vi "CRYStimulus Editor.vi"() -> ()   [LabVIEW 2013]
uses:
  <vilib>/Utility/miscctls.llb/LVBoundsTypeDef.ctl
  Typedef Control/CRYStimulus Cluster.ctl
  Typedef Control/CRYHardware Channel Info.ctl
  Control/CRYStimulusGraphWave.ctl
  CRYProject/CRYProject Editor Global.vi
  SubVI/CRYStimulus Global.vi
  CRYMainGlobal.vi
  CRYWindow/SubVI/CRYMain Sub Window Global.vi
  Program/CRYRef nums global.vi
  CRYStepSetup/CRYStepSetup Global.vi
  CRYSound.dll
panel:
  in  "OkCancelClicked":bool caption="Apply"
  out "Stimulus Bk":T1={"StimulusType"="", "UseMLValArray"=[], "ML_axisArray"=[], "MLValLevelNameArray"=[], "Level(U)Array"=[1.0, 0.0, 0.0, 0.0, 0.0, 0.0, 0.26], "Start(Stop)FreqArray"=[20000.0, 20.0], "Start(Stop)AmpArray"=[0.5, 1.0], "StepResolutionArray"=[], "Unit_Array"=[], "DegValArray"=[], "DegUnitArray"=[], "Steps1"=19, "Cycle/step1(#)"=20, "Time/step1(s)"=0.01, "Transition1"=0.0, "SweepRate2"=1.0, "Freq3(Hz)"=0.0, "Steps3(#)"=19.0, "Cycles3(#)"=12, "StepSize3"=0.0, "wave time"="", "RMS_Value4"=0.0, "Peak_Value4"=0.0, "WavePath4"="", "RMS_unit4"="", "Peak_unit4"="", "wave Info"="", "dc_ctrl5_1"=0, "dc_ctrl5_2"=0, "dc_polar5"=0, "Max.Current"=0, "Steps5(#)"=19, "Time/Step5"=0.05, "Level5"=0.0, "StepsSize5Val"=0.0, "StepSize5Unit"="", "SweepType"=0, "Fixed/Ratio6"=0, "Transition6"=0.0, "Steps6(#)"=19.0, "Cycle/Steps6(#)"=12, "Time/Steps6(s)"=0.0, "Freq6(Hz)"=0.0, "Difference6(Hz)"=0.0, "Ratio6"="", "NoiseType7"=0, "Duration7(s)"=1.0, "MinFreq7(Hz)"=20000.0, "MaxFreq7(Hz)"=20.0, "MinFreq8(Hz)"=20000.0, "MaxFreq8(Hz)"=20.0, "FreqRounding8"=FALSE, "Duration8(s)"=1.0, "Tones8"=0.0, "RoundingVal8"=0.0, "ApplyEQ"=FALSE, "Duration(s)"=0.0, "CustomStimulusName "="", "Flatten Element Array"=[], "sine waves"=[], "Channel Out"=0, "RatioVal6"=0.0, "TabCtrl6"=enum."Master Tone", "Signal Type Name"="", "Help"="", "Channel Sel"=19, "V on DUT"=FALSE, "Output Imp"=6300.0, "Nominal Imp"=100.0} {"Nominal Imp" format="%.2p"; "Output Imp" format="%.2p"; "sine waves"."cycles" format="%.2f"; "sine waves"."ampl" format="%.2f"; "sine waves"."freq" format="%.2f"}
  in  "UpdateTemp":bool caption="Update"
  in  "CurLibChange":bool caption="Add Lib"
  in  "Buffer Index":u32
  in  "Device Name":string
  in  "Asio Limit":u32=16
  in  "Asio Inited":bool caption="Update"
  in  "Audio Driver":u16=16
  in  "Add Lib":bool
  in  "AddStep":bool
  out "Sens Value":dbl
  in  "Help Change":string
  out "EndFlag":bool
  out "Stimulus Play Wave":sgl[](array[numeric])
  out "Is Change?":bool
  in  "Curve Change":enum16{"Curves", "Values", "Results", "WFM"}[](array[ring])
  in  "Channel Out":u32=16
  out "Proper VI No":i32
  out "Signal Type Name":string
  in  "Is First":bool
  in  "Is SubPan?":bool
  out "O_channel Info Out":T2[](array[typedef]) {"Coupling" items=["Default"=-1, "RSE"=10083, "NRSE"=10078, "Differential"=10106, "Pseudodifferential"=12529]; "term config" items=["Default"=-1, "RSE"=10083, "NRSE"=10078, "Differential"=10106, "Pseudodifferential"=12529]; "Anti-aliasing Factor (%fs)" format="%.2f"}
  in  "Vp Out":dbl=2.6 min=0.1 step=0.01 format="%.2f"
  in  "Fs":u32=44100
  in  "BitDepth":u32=16
  in  "Output Device":i16
  in  "ntaskID":u32
  out "Stimulus Wave":sgl[](array[numeric])
  in  "Flatten Element Array":string[](array[string])
  in  "Load Test":bool
  out "Stimulus":T1={"StimulusType"="", "UseMLValArray"=[], "ML_axisArray"=[], "MLValLevelNameArray"=[], "Level(U)Array"=[1.0, 0.0, 0.0, 0.0, 0.0, 0.0, 0.26], "Start(Stop)FreqArray"=[20000.0, 20.0], "Start(Stop)AmpArray"=[0.5, 1.0], "StepResolutionArray"=[], "Unit_Array"=[], "DegValArray"=[], "DegUnitArray"=[], "Steps1"=19, "Cycle/step1(#)"=20, "Time/step1(s)"=0.01, "Transition1"=0.0, "SweepRate2"=1.0, "Freq3(Hz)"=0.0, "Steps3(#)"=19.0, "Cycles3(#)"=12, "StepSize3"=0.0, "wave time"="", "RMS_Value4"=0.0, "Peak_Value4"=0.0, "WavePath4"="", "RMS_unit4"="", "Peak_unit4"="", "wave Info"="", "dc_ctrl5_1"=0, "dc_ctrl5_2"=0, "dc_polar5"=0, "Max.Current"=0, "Steps5(#)"=19, "Time/Step5"=0.05, "Level5"=0.0, "StepsSize5Val"=0.0, "StepSize5Unit"="", "SweepType"=0, "Fixed/Ratio6"=0, "Transition6"=0.0, "Steps6(#)"=19.0, "Cycle/Steps6(#)"=12, "Time/Steps6(s)"=0.0, "Freq6(Hz)"=0.0, "Difference6(Hz)"=0.0, "Ratio6"="", "NoiseType7"=0, "Duration7(s)"=1.0, "MinFreq7(Hz)"=20000.0, "MaxFreq7(Hz)"=20.0, "MinFreq8(Hz)"=20000.0, "MaxFreq8(Hz)"=20.0, "FreqRounding8"=FALSE, "Duration8(s)"=1.0, "Tones8"=0.0, "RoundingVal8"=0.0, "ApplyEQ"=FALSE, "Duration(s)"=0.0, "CustomStimulusName "="", "Flatten Element Array"=[], "sine waves"=[], "Channel Out"=0, "RatioVal6"=0.0, "TabCtrl6"=enum."Master Tone", "Signal Type Name"="", "Help"="", "Channel Sel"=19, "V on DUT"=FALSE, "Output Imp"=6300.0, "Nominal Imp"=100.0} {"Nominal Imp" format="%.2p"; "Output Imp" format="%.2p"; "sine waves"."cycles" format="%.2f"; "sine waves"."ampl" format="%.2f"; "sine waves"."freq" format="%.2f"}
  in  "All Parameter Change":bool
  out "VIMiniumBound":T3
  in  "Channel":i32
  in  "Calibration setup In":string
  in  "Hardware setup In":string
  out "Flatten Stimulus Out":string
  in  "reference out":refnum<vi>
  in  "stop":bool
  in  "Board Tab":enum32{"Page 1"}(tab) caption="Control Tab"
  in  "Progress":string
  in  "Apply EQ":bool caption="使用均衡器"
  in  "Custom Stimulus Name":string caption="自定义激励名称"
  out "Duration(s)":dbl caption="持续时间(s)" format="%#_6p"
  in  "Update":bool
  in  "Play":bool
  in  "Output Channel":bool
  in  "ViewTable":bool
  in  "Table Tab":enum32{"Setting", "Help"}(tab)
  in  "Move Down":bool
  in  "Move Up":bool
  in  "Remove":bool
  in  "Insert":bool
  in  "Edit":bool
  in  "Multicolumn Listbox":i32(listbox)
  in  "Help":string
  in  "delta_str":string
  in  "delta_X":dbl format="%#.3p"
  in  "delta_Y":dbl
  in  "View Edit":bool
  out "Wave graph":T4
  in  "Buf Amount":u32=16
  out "Stim max value":sgl
  in  "Revert":bool caption="Apply"
  in  "Load...":bool caption="Apply"
  in  "Save As...":bool caption="Apply"
  in  "OK":bool caption="Apply"
  in  "Cancel":bool caption="Apply"
  # "(1,2,3,4,6_1,6_2,7,8)"
  # "(1,2,3,4,6_1,6_2,7,8)"
  # "(1,2,3,4,6_1,6_2,7,8)"
  # "(1,2,4,6_1,6_2,7,8)"
  # "(1,2,6)"
  # "(3,5)"
  # "(1,6,8)"
  # "(1,2,4,6_1,6_2,7,8)"
  # "(1,2,3,4,6_1,6_2,7,8)"
  # "(1,2,3,4,6_1,6_2,7,8)"
  # "(1,2,3,4,6_1,6_2,7,8)"
  # "(1,2,3,4,6_1,6_2,7,8)"
  # "(1,2,3,4,6_1,6_2,7,8)"
  # "(1,2,4,6_1,6_2,7,8)"
  # "(1,2,6)"
  # "(3,5)"
  # "(1,6,8)"
  # "(1,2,4,6_1,6_2,7,8)"
  # "(1,2,3,4,6_1,6_2,7,8)"
  # "(1,2,3,4,6_1,6_2,7,8)"
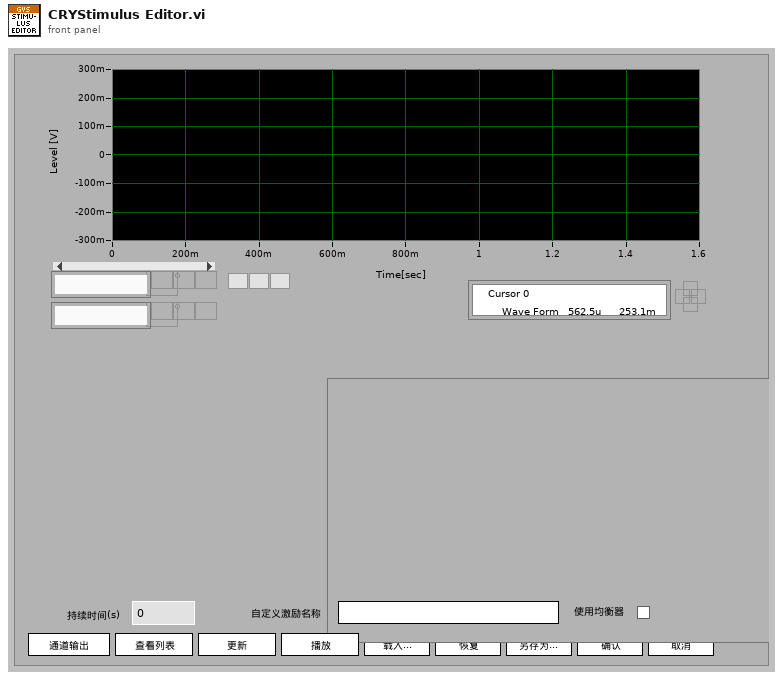
[diagram p1: front panel]
types:
  T1 = typedef "CRYStimulus Cluster.ctl" = cluster{"StimulusType":string, "UseMLValArray":u16[], "ML_axisArray":u16[], "MLValLevelNameArray":string[], "Level(U)Array":dbl[], "Start(Stop)FreqArray":dbl[], "Start(Stop)AmpArray":dbl[], "StepResolutionArray":u16[], "Unit_Array":u16[], "DegValArray":dbl[], "DegUnitArray":string[], "Steps1":i32, "Cycle/step1(#)":u32, "Time/step1(s)":dbl, "Transition1":dbl, "SweepRate2":dbl, "Freq3(Hz)":dbl, "Steps3(#)":dbl, "Cycles3(#)":u32, "StepSize3":dbl, "wave time":string, "RMS_Value4":dbl, "Peak_Value4":dbl, "WavePath4":string, "RMS_unit4":string, "Peak_unit4":string, "wave Info":string, "dc_ctrl5_1":u16, "dc_ctrl5_2":u16, "dc_polar5":u16, "Max.Current":u16, "Steps5(#)":u32, "Time/Step5":dbl, "Level5":dbl, "StepsSize5Val":dbl, "StepSize5Unit":string, "SweepType":u16, "Fixed/Ratio6":u16, "Transition6":dbl, "Steps6(#)":dbl, "Cycle/Steps6(#)":u32, "Time/Steps6(s)":dbl, "Freq6(Hz)":dbl, "Difference6(Hz)":dbl, "Ratio6":string, "NoiseType7":u16, "Duration7(s)":dbl, "MinFreq7(Hz)":dbl, "MaxFreq7(Hz)":dbl, "MinFreq8(Hz)":dbl, "MaxFreq8(Hz)":dbl, "FreqRounding8":bool, "Duration8(s)":dbl, "Tones8":dbl, "RoundingVal8":dbl, "ApplyEQ":bool, "Duration(s)":dbl, "CustomStimulusName ":string, "Flatten Element Array":string[], "sine waves":cluster{"freq":dbl, "ampl":dbl, "cycles":dbl}[], "Channel Out":i32, "RatioVal6":dbl, "TabCtrl6":enum32{"Master Tone", "Slave Tone"}, "Signal Type Name":string, "Help":string, "Channel Sel":u16, "V on DUT":bool, "Output Imp":dbl, "Nominal Imp":dbl}
  T2 = typedef "CRYHardware Channel Info.ctl" = cluster{"ID":i32, "Name":string, "Digital":bool, "Input":bool, "Device Name":string, "Hardware Ch ID":u8, "Vmax (V)":dbl, "Latency (samples)":dbl, "Sampling Rate (Hz)":u32, "Bit Depth":u32, "Anti-aliasing Factor (%fs)":sgl, "DAQmx Channel":tag, "term config":i32, "Coupling":i32, "IEPE en":bool, "ASIOChannel Name":string, "Audio Driver":u16, "ASIOChannel Index":u8}
  T3 = typedef "LVBoundsTypeDef.ctl" = cluster{"Width":u32, "Height":u32}
  T4 = typedef "CRYStimulusGraphWave.ctl" = waveform(dbl)
  T5 = cluster{"halt now":bool, "exit":bool, "dll done":bool, "Hardware":i32, "start":bool}
  T6 = typedef "CRYHardware.ctl" = cluster{"Name":string, "Analog I/O":u16, "Digital I/O":u16, "Channels":u8, "Dig Dev ID":u8, "N ports":u8, "Interface":u32, "Dig I/O Ports":cluster{"port #":i16, "width":i16, "direction":i32}[], "Interf settings":cluster{"Type":u16, "COM Port":u8, "Baud rate":u32, "Data bits":u32, "Parity":u16, "Stop bits":u16, "Flow control":u16, "Dev ID IEEE":u8}[], "N interfs":i32, "udev SNs":i16[], "udev enable":bool, "Channel Array":T2[], "Cal sequence":string, "SelectedIn":u16, "SelectedOut":u16, "SelectedTab":u16, "State":bool, "Help":string, "Advanced":bool, "In Audio Driver":u16, "Out Audio Driver":u16}
  T7 = typedef "CRYCalibration All Cluster.ctl" = cluster{"Calibration 2D":T8[], "Help":string, "Tab Value":i32, "Input Signal Type":string, "Output Signal Type":string}
  T8 = typedef "CRYCalibration 2DCluster.ctl" = cluster{"Calibration":T9, "Corr Curve":T10, "EQ Curve":T10, "Sens Curve":T10}
  T9 = typedef "CRYCalibration Cluster.ctl" = cluster{"Calibration Step Name":string, "Device":string, "Correction Curve Name":string, "Equalization Curve Name":string, "Sensitivity Curve Name":string, "Corr Folder and File":string, "EQ Folder and File":string, "Sens Folder and File":string, "Corr Step size":u16, "EQ Step size":u16, "Input":bool, "Last Cal Date (sec)":timestamp, "Cha Name":string, "Corr Curve Found":bool, "EQ Curve Found":bool, "Sens Curve Found":bool, "Signal Type":string, "Calibrated Device":string, "Hz":u32}
  T10 = typedef "CRYData Cluster.ctl" = cluster{"Name":string, "Curve":cluster{"x":dbl, "y":dbl, "z":dbl}[], "X data":u16, "Y data":u16, "Z data":u16, "X axis":u16, "Y axis":u16, "Z axis":u16, "X unit":string, "Y unit":string, "Z unit":string, "X dB ref":dbl, "Y dB ref":dbl, "Z dB ref":dbl, "single val":bool, "protected":bool, "display X":bool, "display Y":bool, "display Z":bool, "Test Info":string, "Step No.":i32, "Plot Settings":cluster{"Color":u32, "Interpolation":u8, "Point Style":u8, "Line Style":u8, "Point Color":u32, "Line Width":u8, "Bar Plot Style":u8, "Fill To":i16}, "AutoProtect":bool}
  T11 = typedef "CRYStep.ctl" = cluster{"No.VI":i32, "Category":string, "StepName":string, "Seq setup flattened":string, "Comment":string, "Steps config.":bool[], "Jump config":i32[], "Start":dbl, "Increment":dbl, "Name":string, "Unit":string, "Y data":u16, "Y prefix":string, "Y dB ref":dbl, "Y unit":string, "Repeat State Array":cluster{"Start":dbl, "Increment":dbl, "Count":i32, "Num":i32}[]}
  T12 = enum8{"Enabled", "Disabled", "Disabled and Grayed Out"}
  T13 = enum32{"Invalid", "Default", "Floating", "Floating/Auto-Hide", "Modal"}
  T14 = enum16{"OK", "Yes", "YesNo", "YesNoCancel", "ReplaceAppend"}
  T15 = typedef "CRYWaveform Cluster.ctl" = cluster{"Waveform":cluster{"X0":dbl, "dX":dbl, "Y":sgl[]}, "X data":u16, "Y data":u16, "Y axis":u16, "X unit":string, "Y unit":string, "Y dB ref":dbl, "display Y":bool, "display X":bool, "Overload?":bool, "Test Info":string, "Step No.":i32, "Name":string, "protected":bool, "Sqc history":string[], "Signal Channel ID":i32, "Plot Settings":cluster{"Color":u32, "Interpolation":u8, "Point Style":u8, "Line Style":u8, "Point Color":u32, "Line Width":u8, "Bar Plot Style":u8, "Fill To":i16}, "AutoProtect":bool}
  T16 = cluster{"Load Test":bool, "Output Channel":bool, "Edit":bool, "Insert":bool, "Remove":bool, "Move Up":bool, "Move Down":bool, "ViewTable":bool, "View Edit":bool, "Add Lib":bool, "OK":bool, "Cancel":bool}
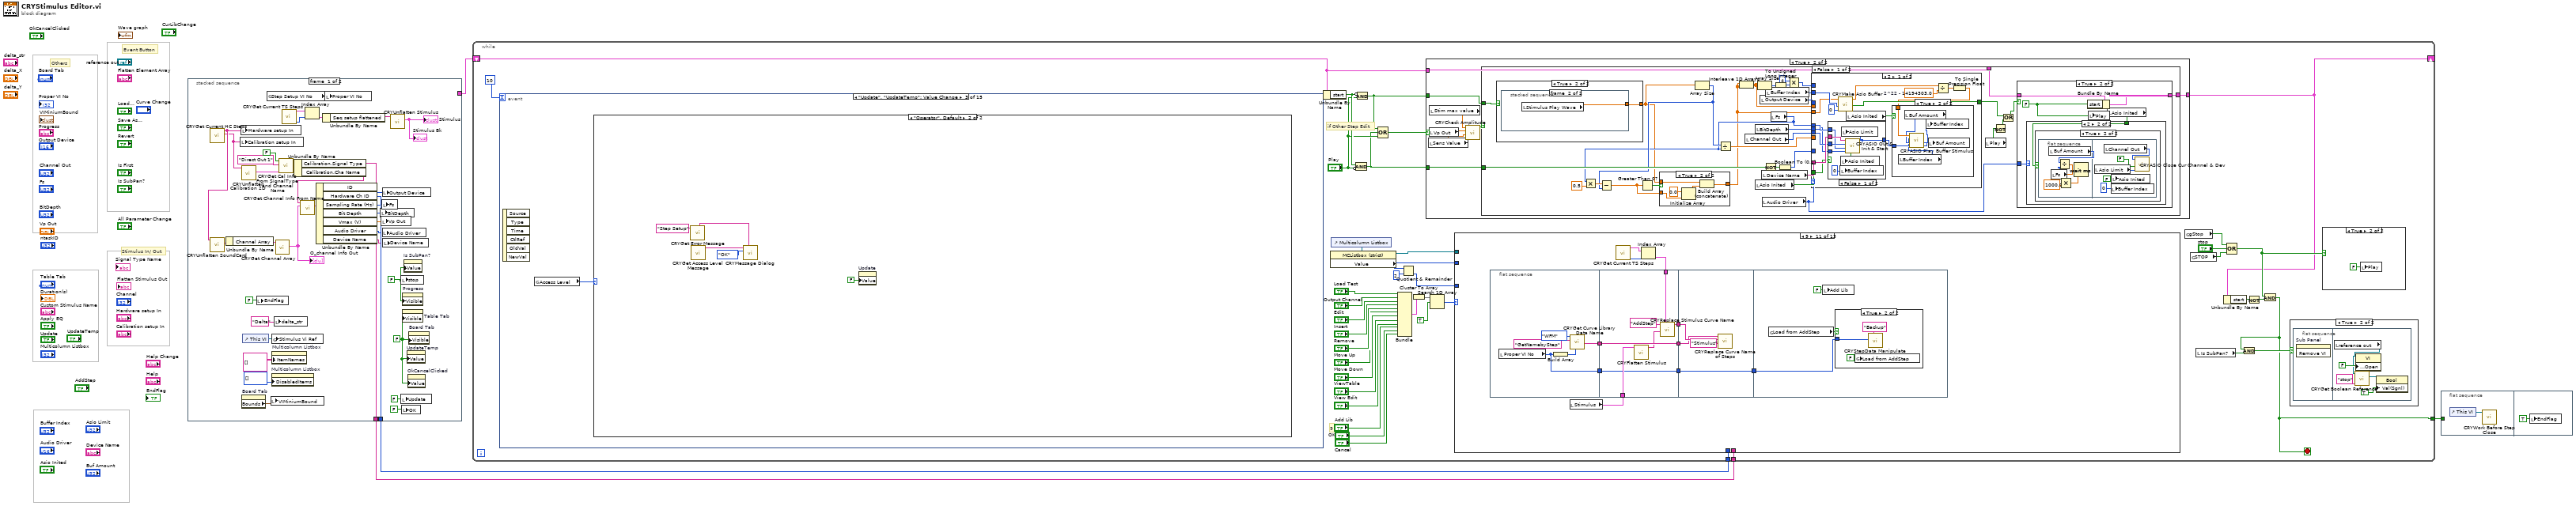
[diagram p0: block diagram]
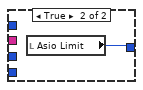
[diagram p6: hidden frame]
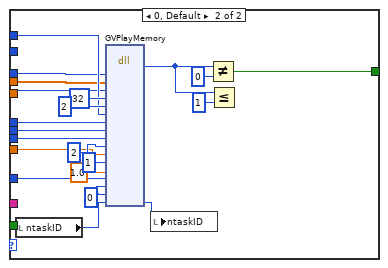
[diagram p7: hidden frame]
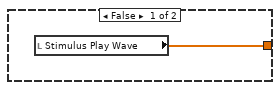
[diagram p9: hidden frame]
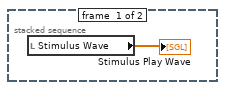
[diagram p10: hidden frame]
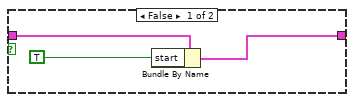
[diagram p11: hidden frame]
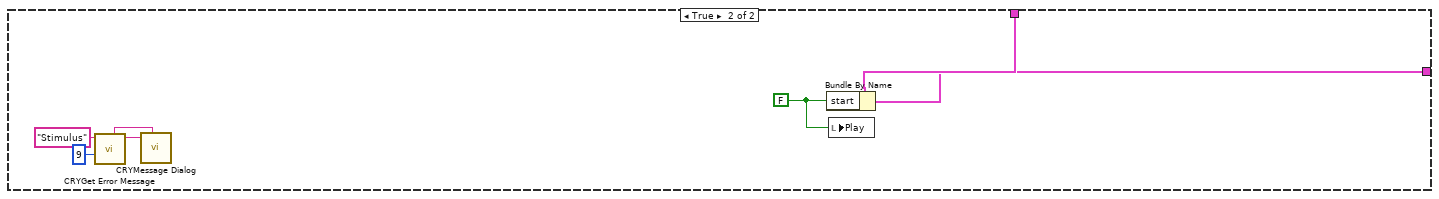
[diagram p14: hidden frame]
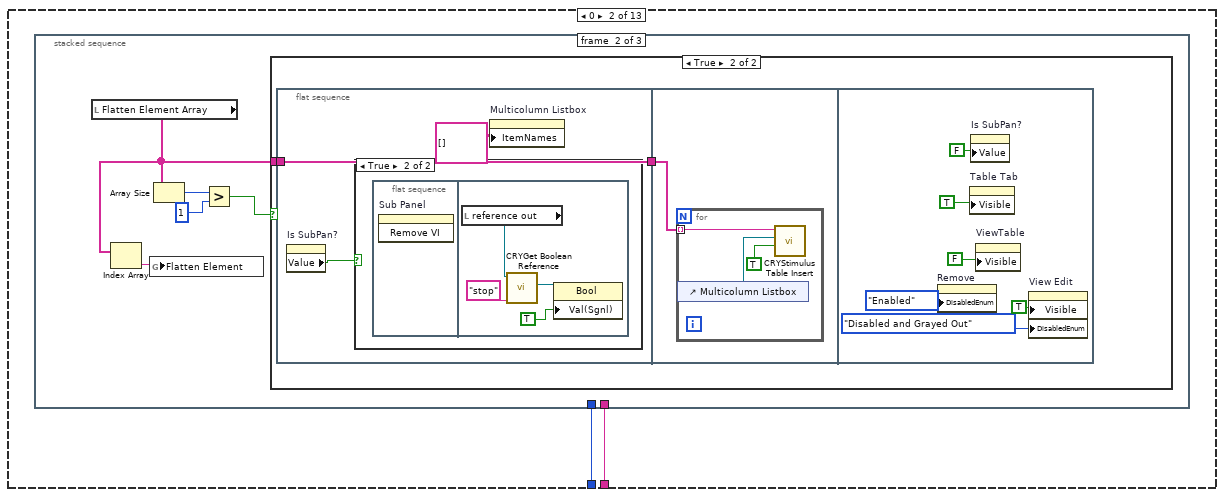
[diagram p16: hidden frame]
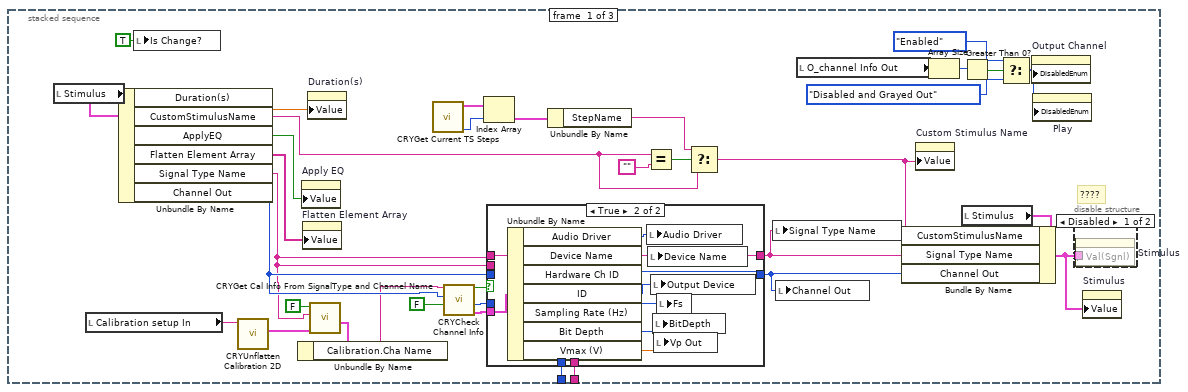
[diagram p17: hidden frame]
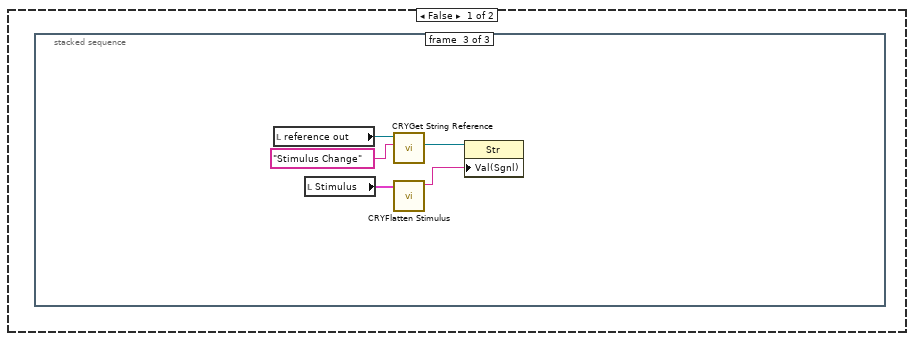
[diagram p20: hidden frame]
diagram:
  # "Others"
  # "Event Button"
  # "Stimulus In/ Out"
  n1 = stacked-sequence {
    tunnel: [_ T5 {"halt now"=FALSE, "exit"=FALSE, "dll done"=FALSE, "Hardware"=-1, "start"=FALSE}] -> w4
    tunnel: [w14 _] -> w2
    tunnel: [w23 _] -> w3
    frame #0 {
      w7 = FALSE ("Visible")
      w27 = FALSE ("Visible")
      n2 = call "CRYGet Current HC Steps.vi"() -> ("Calibration setup flattened Out"=w19:string, "Hardware setup flattened Out"=w20:string)  [unwired: 10 in]
      n3 = call "CRYUnflatten SoundCard.vi"("Flatten SoundCard"=w20) -> ("SoundCard"=w33:T6)  [unwired: 10 out]
      n4 = Unbundle By Name(w33) -> ("Channel Array"=w34:T2[])
      n5 = local write "Calibration setup In"(w19) -> ()
      n6 = local write "Hardware setup In"(w20) -> ()
      n7 = call "CRYUnflatten Calibration 2D.vi"("Flattened Calibration"=w19) -> ("Calibration Step Out"=w18:T7)  [unwired: 8 in, 2 out]
      n8 = property on="Board Tab" class="TabCtl (strict)"() -> ("Bounds"=w38:T3)  [unwired: 2 in, 2 out]
      n9 = control-ref of="This VI"() -> (w28:refnum<vi>)
      n10 = local write "EndFlag"(FALSE ("endflag")) -> ()
      n11 = global read "CRYProject Editor Global.vi" "Step Setup VI No"() -> (w39:i32)
      n12 = local write "VIMiniumBound"(w38) -> ()
      n13 = global write "CRYStimulus Global.vi" "Stimulus Vi Ref"(w28) -> ()
      n14 = property on="Multicolumn Listbox" class="MCListbox (strict)"("DisabledItems"=i32[] [] ("Disabled Items")) -> ()  [unwired: 2 in, 2 out]
      n15 = property on="Multicolumn Listbox" class="MCListbox (strict)"("ItemNames"=string[][] [] ("Item Names")) -> ()  [unwired: 2 in, 2 out]
      n16 = local write "delta_str"("Delta" ("delta_str")) -> ()
      n17 = call "CRYGet Channel Array.vi"("Channel Array"=w34) -> ("O Channel Info Out"=w13:T2[])  [unwired: 10 out]
      "O_channel Info Out" <- w13
      n18 = call "CRYGet Cal Info From SignalType and Channel Name.vi"("Calibration"=w18, "Signal Type"="Direct Out 1" ("Calibration.Signal Type"), "In/Out?"=FALSE) -> ("Calibration 2D Cluster"=w15:T8)  [unwired: 6 in, 2 out]
      n19 = call "CRYGet Current TS Steps.vi"() -> ("SelectStepNumber in Tree"=w25:i32, "Steps"=w26:T11[])  [unwired: 1 in, 9 out]
      n20 = Unbundle By Name(w15) -> ("Calibration.Signal Type"=w14:string, "Calibration.Cha Name"=w12:string)
      n21 = call "CRYGet Channel Info From Name.vi"("Channel Info Array In"=w13, "Channel Name"=w12) -> ("ChannelInfo"=w11:T2)  [unwired: 8 in, 1 out]
      n22 = Index Array(array=w26, index=w25) -> (element=w35:T11)
      n23 = Unbundle By Name(w11) -> ("ID"=w29:i32, "Hardware Ch ID"=w23:u8, "Sampling Rate (Hz)"=w30:u32, "Bit Depth"=w32:u32, "Vmax (V)"=w31:dbl, "Audio Driver"=w10:u16, "Device Name"=w9:string)
      n24 = Unbundle By Name(w35) -> ("Seq setup flattened"=w36:string)
      n25 = local write "Proper VI No"(w39) -> ()
      n26 = local write "BitDepth"(w32) -> ()
      n27 = local write "Vp Out"(w31) -> ()
      n28 = local write "Fs"(w30) -> ()
      n29 = local write "Output Device"(w29) -> ()
      n30 = local write "Audio Driver"(w10) -> ()
      n31 = local write "Device Name"(w9) -> ()
      n32 = call "CRYUnflatten Stimulus.vi"("Flatten Stimulus"=w36) -> ("Stimulus"=→"Stimulus" →"Stimulus Bk":T1)  [unwired: 10 out]
      n33 = local write "stop"(w27) -> ()
      n34 = local write "Update"(FALSE ("Update")) -> ()
      n35 = local write "OK"(FALSE ("OK")) -> ()
      n36 = property on="Table Tab" class="TabCtl (strict)"("Visible"=w7) -> ()  [unwired: 2 in, 2 out]
      n37 = property on="Progress" class="Str"("Visible"=w27) -> ()  [unwired: 2 in, 2 out]
      n38 = property on="Is SubPan?" class="Bool (strict)"("Value"=w27) -> ()  [unwired: 2 in, 2 out]
      n39 = property on="UpdateTemp" class="Bool (strict)"("Value"=w7) -> ()  [unwired: 2 in, 2 out]
      n40 = property on="OkCancelClicked" class="Bool (strict)"("Value"=w7) -> ()  [unwired: 2 in, 2 out]
      n41 = property on="Board Tab" class="TabCtl (strict)"("Visible"=w7) -> ()  [unwired: 2 in, 2 out]
    }
    frame #1 {
      w41 = TRUE ("Load Test")
      n42 = local write "Stimulus Play Wave"(sgl[] [] ("Stimulus Play Wave")) -> ()
      n43 = local write "Is Change?"(w41) -> ()
      n44 = local write "Load Test"(w41) -> ()
      n45 = property on="Is First" class="Bool (strict)"("Value"=w41) -> ()  [unwired: 2 in, 2 out]
    }
  }
  n46 = while {
    shift-right: [w45] -> _
    shift-left: w4 -> [w75]
    tunnel: w3 -> [w52]
    tunnel: w2 -> [w53]
    tunnel: [w48] -> w1
    stop <- w48 stop-if-true
    # "9"
    # "if Other Step Edit"
    n47 = event shown="[2] \"Update\", \"UpdateTemp\": Value Change" {
      selector: _ -> [_ _ _ _ _ _ _ _ _ _ _ _ _ _ _]
      dyn-events: _ -> [_ _ _ _ _ _ _ _ _ _ _ _ _ _ _]
      timeout: 10 -> [_ _ _ _ _ _ _ _ _ _ _ _ _ _ _]
      event Timeout {
        n48 = event-data() -> ()  [unwired: 3 out]
      }
      event Pane Size {
        n49 = event-data() -> ()  [unwired: 7 out]
        n50 = control-ref of="Board Tab"() -> (w673:refnum<vi>)
        n51 = control-ref of="This VI"() -> (w674:refnum<vi>)
        n52 = call "CRYAlign Steps VI Center.vi"("Tab2"=w673, "Input/Output"=TRUE, "VIRef"=w674) -> ()  [unwired: 1 in, 8 out]
      }
      event "Update", "UpdateTemp": Value Change {
        n53 = event-data() -> ()  [unwired: 7 out]
        n54 = global read "CRYMainGlobal.vi" "Access Level"() -> (w676:enum16{"Engineer", "Technician", "Operator"})
        n55 = case shown="\"Operator\", Default" w676 {
          frame "Engineer" {
            n56 = property on="Table Tab" class="TabCtl (strict)"() -> ("Visible"=w678:bool)  [unwired: 2 in, 2 out]
            n57 = property on="Is First" class="Bool (strict)"() -> ("Value"=w679:bool)  [unwired: 2 in, 2 out]
            n58 = case shown="False" w678 {
              tunnel: w679 -> [w681 _]
              tunnel: [w680 w705] -> w677
              frame False {
                n59 = case shown="False" w681 {
                  tunnel: [w685 TRUE ("Error")] -> w680
                  frame False {
                    w690 = TRUE ("Is SubPan?")
                    n60 = local read "Flatten Element Array"() -> (w688:string[])
                    n61 = global read "CRYStimulus Global.vi" "Flatten Element"() -> (w689:string)
                    n62 = local read "Is Change?"() -> (w683:bool)
                    n63 = Index Array(array=w688) -> (element=w687:string)  [unwired: 1 in]
                    n64 = call "CRYCheck Change Before Update.vi"("New Flatten Stimulus Element"=w689, "Old Flatten Stimulus Element"=w687) -> ("Is Change?"=w684:bool)  [unwired: 9 out]
                    n65 = call "CRYCheck EditVal.vi"("Is SubPan?"=w690, "display message?"=w690, "Flatten Element"=w689) -> ("Error"=w686:bool)  [unwired: 1 in, 7 out]
                    n66 = Or(x=w684, y=w683) -> (x .or. y?=w682:bool)
                    n67 = Compound Arithmetic op=AND(invert w686, w682) -> (w685:bool)
                    n68 = case shown="True" w685 {
                      tunnel: w689 -> [_ w692]
                      tunnel: w688 -> [_ w691]
                      frame False {
                      }
                      frame True {
                        n69 = Array Size(array=w691) -> (size(s)=w695:i32)
                        n70 = Equal To 0?(x=w695) -> (x = 0?=w694:bool)
                        n71 = case shown="False" w694 {
                          tunnel: w691 -> [w699 w702]
                          tunnel: w692 -> [w698 w701]
                          tunnel: [w696 w700] -> w693
                          frame False {
                            n72 = Replace Array Subset(array=w699, new element=w698, index=0) -> (w696:string[])
                          }
                          frame True {
                            n73 = Insert Into Array(array=w702, index=0, new element=w701) -> (w700:string[])
                          }
                        }
                        n74 = property on="Flatten Element Array" class="Arr (strict)"("Value"=w693) -> ()  [unwired: 2 in, 2 out]
                      }
                    }
                  }
                  frame True {
                  }
                }
              }
              frame True {
                n75 = control-ref of="Multicolumn Listbox"() -> (w708:refnum<vi>)
                n76 = local read "Is Change?"() -> (w706:bool)
                n77 = call "CRYCheck EditVal.vi"("Is SubPan?"=FALSE, "display message?"=TRUE, "MCListbox Refnum"=w708) -> ("Error"=w707:bool)  [unwired: 1 in, 7 out]
                n78 = Compound Arithmetic op=AND(invert w707, w706) -> (w705:bool)
              }
            }
            n79 = case shown="True" w677 {
              frame False {
                n80 = property on="Update" class="Bool (strict)"("Value"=FALSE ("Update")) -> ()  [unwired: 2 in, 2 out]
              }
              frame True {
                n81 = stacked-sequence {
                  seq-local: [_ w718 _ _] -> [_ _ w741 _]
                  frame #0 {
                    n82 = control-ref of="Progress"() -> (w714:refnum<vi>)
                    n83 = call "CRYGet Error Message.vi"("Error No"=2, "Kind"="Stimulus") -> ("Unicode Message"=w712:string)  [unwired: 4 in, 5 out]
                    n84 = property on="Progress" class="Str"("Visible"=TRUE) -> ()  [unwired: 2 in, 2 out]
                    n85 = call "CRYDisplay Unicode String Text.vi"("Interpret as Unicode (T)"=TRUE, "String Value"=w712, "String Control Reference"=w714) -> ()  [unwired: 5 in, 2 out]
                  }
                  frame #1 {
                    n86 = property on="Is First" class="Bool (strict)"() -> ("Value"=w729:bool)  [unwired: 2 in, 2 out]
                    n87 = property on="Is SubPan?" class="Bool (strict)"() -> ("Value"=w730:bool)  [unwired: 2 in, 2 out]
                    n88 = local read "Stimulus"() -> (w726:T1)
                    n89 = Not(x=w729) -> (.not. x?=w728:bool)
                    n90 = And(x=w730, y=w728) -> (x .and. y?=w727:bool)
                    n91 = case shown="True" w727 {
                      tunnel: w726 -> [w731 w733]
                      tunnel: [w731 w732] -> w719
                      frame False {
                      }
                      frame True {
                        n92 = local read "reference out"() -> (w735:refnum<vi>)
                        n93 = invoke class="VI" method="Ctrl Val.Get"(reference=w735, "Control Name"="Stimulus Out") -> ("Get Control Value Variant"=w734:variant)  [unwired: 2 in, 3 out]
                        n94 = Variant To Data(type=w733, Variant=w734) -> (data=w732:T1)  [unwired: 1 in, 1 out]
                      }
                    }
                    n95 = local read "Signal Type Name"() -> (w720:string)
                    n96 = local read "Channel Out"() -> (w721:u32)
                    n97 = property on="Duration(s)" class="DigNum (strict)"() -> ("Value"=w723:dbl)  [unwired: 2 in, 2 out]
                    n98 = property on="Custom Stimulus Name" class="Str"() -> ("Value"=w722:string)  [unwired: 2 in, 2 out]
                    n99 = property on="Apply EQ" class="Bool (strict)"() -> ("Value"=w724:bool)  [unwired: 2 in, 2 out]
                    n100 = local read "Flatten Element Array"() -> (w725:string[])
                    n101 = Bundle By Name(cluster=w719, "Flatten Element Array"=w725, "Duration(s)"=w723, "CustomStimulusName"=w722, "ApplyEQ"=w724, "Channel Out"=w721, "Signal Type Name"=w720) -> (w718:T1)
                    n102 = local write "Stimulus"(w718) -> ()
                  }
                  frame #2 {
                    n103 = local read "Proper VI No"() -> (w740:i32)
                    n104 = local read "Flatten Element Array"() -> (w745:string[])
                    n105 = Array Size(array=w745) -> (size(s)=w744:i32)
                    n106 = Build Array(w740) -> (w739:i32[])
                    n107 = call "CRYGet Curve Library Data Name.vi"("nData"=w739, "sAction"="GetNamebyStep" ("sOption")) -> ("sNames"=w737:string[])  [unwired: 6 in, 3 out]
                    n108 = Greater Than 0?(x=w744) -> (x > 0?=w742:bool)
                    n109 = case shown="True" w742 {
                      tunnel: w745 -> [_ _]
                      tunnel: [0.0 w758] -> w743
                      tunnel: w741 -> [_ w779]
                      tunnel: w737 -> [_ w759]
                      frame False {
                      }
                      frame True {
                        w752 = 4194303.0  # 2^22 - 1
                        # "?????????"
                        n110 = Unbundle By Name(w779) -> ("Signal Type Name"=w778:string)
                        n111 = local read "Stimulus"() -> (w769:T1)
                        n112 = local read "Calibration setup In"() -> (w761:string)
                        n113 = local read "Hardware setup In"() -> (w762:string)
                        n114 = call "CRYGet Current TS Steps.vi"() -> ("SelectStepNumber in Tree"=w771:i32, "Steps"=w770:T11[])  [unwired: 1 in, 9 out]
                        n115 = call "CRYGet Current Calibration Info.vi"("Is Input?"=FALSE, "Signal Type Name"=w778) -> ("Calibration All Cluster"=w784:T8)  [unwired: 9 out]
                        n116 = call "CRYFlatten Stimulus.vi"("Stimulus"=w769) -> ("Flatten Stimulus String"=w767:string)  [unwired: 10 in]
                        n117 = Index Array(array=w770, index=w771) -> (element=w768:T11)
                        n118 = Unbundle By Name(w784) -> ("Sens Curve"=w787:T10)
                        n119 = Bundle By Name(cluster=w768, "Seq setup flattened"=w767) -> (w763:T11)
                        n120 = call "CRYStimulus.vi"("Setup in"=w763, "Hardware in"=w762, "Calibration in"=w761) -> ("Inserted Names Out"=w760:string[], "Wave out"=w764:T15[])  [unwired: 8 in, 3 out]
                        n121 = Unbundle By Name(w787) -> ("Y unit"=w783:string, "Curve"=w774:cluster{"x":dbl, "y":dbl, "z":dbl}[], "Y dB ref"=w773:dbl, "Y data"=w772:u16)
                        n122 = Index Array(array=w764) -> (element=w788:T15)  [unwired: 1 in]
                        n123 = local read "Fs"() -> (w755:u32)
                        n124 = Unbundle By Name(w788) -> ("Waveform.Y"=w750:sgl[])
                        n125 = Index Array(array=w774) -> (element=w791:cluster{"x":dbl, "y":dbl, "z":dbl})  [unwired: 1 in]
                        n126 = Reciprocal(x=w755) -> (1/x=w756:dbl)
                        n127 = Unbundle By Name(w791) -> ("y"=w775:dbl)
                        n128 = Match Pattern(string=w783, regular expression="/") -> (before substring=w782:string)  [unwired: 4 out]
                        n129 = case shown="0, Default" w772 {
                          tunnel: w775 -> [w802 w803]
                          tunnel: [w801 w803] -> w776
                          tunnel: w773 -> [w800 _]
                          frame 0, Default {
                            n130 = call "CRYConversion dB-Lin.vi"("dB ref."=w800, "Log In"=w802) -> ("Lin Out"=w801:dbl)  [unwired: 4 in, 3 out]
                          }
                          frame 1 {
                          }
                        }
                        n131 = disable-structure shown="Disabled" {
                          disable-tunnel: w760 -> [w793 w795]
                          disable-tunnel: w759 -> [w792 w796]
                          frame Disabled {
                            n132 = call "CRYReplace Curve Name of Steps.vi"("Step Category"="Stimulus", "New Name"=w793, "Old Name"=w792) -> ()  [unwired: 8 in, 1 out]
                          }
                          frame Enabled {
                            n133 = call "CRYChange Name by Step Editor.vi"("Old Names"=w796, "New Names"=w795) -> ()  [unwired: 10 in]
                          }
                        }
                        n134 = Concatenate Strings("Level [" ("string"), w782, "]" ("string")) -> (w765:string)
                        n135 = Array Max & Min(array=w750) -> (max value=→"Stim max value":sgl)  [unwired: 3 out]
                        n136 = Array Size(array=w750) -> (size(s)=w757:i32)
                        n137 = Bundle By Name("Y"=w750, "dt"=w756) -> (w766:waveform(sgl))  [unwired: 1 out]
                        n138 = property on="Wave graph" class="WFGraph (strict)"("YScale.NameLbl.Text"=w765) -> ()  [unwired: 2 in, 2 out]
                        n139 = Multiply(x=w757, y=w756) -> (x*y=w758:dbl)
                        n140 = local read "Vp Out"() -> (w754:dbl)
                        n141 = Less Than 0?(x=w776) -> (x < 0?=w790:bool)
                        n142 = local write "Sens Value"(w776) -> ()
                        n143 = stacked-sequence {
                          tunnel: w766 -> [w797 _]
                          frame #0 {
                            n144 = local write "Wave graph"(w797) -> ()
                          }
                          frame #1 {
                            n145 = control-ref of="Wave graph"() -> (w799:refnum<vi>)
                            n146 = call "CRYPaint WaterMark.vi"("Type"="Small", "Graph Ref"=w799) -> ()  [unwired: 10 in]
                          }
                        }
                        n147 = Select(t=1.0, s=w790, f=w776) -> (s? t:f=w753:dbl)
                        n148 = Multiply(x=w753, y=w754) -> (x*y=w749:dbl)
                        n149 = Divide(x=w752, y=w749) -> (x/y=w747:dbl)
                        n150 = To Single Precision Float(number=w747) -> (single precision float=w751:sgl)
                        n151 = Multiply(x=w750, y=w751) -> (x*y=→"Stimulus Wave":sgl[])
                      }
                    }
                    n152 = local write "Duration(s)"(w743) -> ()
                  }
                  frame #3 {
                    w805 = FALSE ("Is First")
                    # "Insert Curves Library."
                    n153 = property on="Update" class="Bool (strict)"("Value"=FALSE ("Update")) -> ()  [unwired: 2 in, 2 out]
                    n154 = property on="Is First" class="Bool (strict)"("Value"=w805) -> ()  [unwired: 2 in, 2 out]
                    n155 = local write "Is Change?"(w805) -> ()
                    n156 = property on="Progress" class="Str"("Visible"=FALSE) -> ()  [unwired: 2 in, 2 out]
                  }
                }
              }
            }
          }
          frame "Operator", Default {
            n157 = call "CRYGet Error Message.vi"("Kind"="Step Setup") -> ("Window Title"=w808:string)  [unwired: 5 in, 5 out]
            n158 = call "CRYGet Access Level Message.vi"() -> ("Multibyte string"=w810:string)  [unwired: 11 in]
            n159 = call "CRYMessage Dialog.vi"("Window Title"=w808, "YesNoCancel"=T14."OK", "Message Content"=w810) -> ()  [unwired: 7 in, 2 out]
            n160 = property on="Update" class="Bool (strict)"("Value"=FALSE ("Update")) -> ()  [unwired: 2 in, 2 out]
          }
        }
      }
      event "Save As...": Value Change {
        n161 = event-data() -> ("CtlRef"=w812:refnum<vi>)  [unwired: 6 out]
        n162 = property class="Bool (strict)"(reference=w812, "Value"=FALSE) -> ()  [unwired: 1 in, 2 out]
        n163 = local read "Stimulus"() -> (w814:T1)
        n164 = global read "CRYMainGlobal.vi" "Steps path"() -> (w816:path)
        n165 = local read "Proper VI No"() -> (w823:i32)
        n166 = call "CRYFlatten Stimulus.vi"("Stimulus"=w814) -> ("Flatten Stimulus String"=w820:string)  [unwired: 10 out]
        n167 = Build Path(base path=w816, name or relative path="CRYStimulus") -> (appended path=w815:path)
        n168 = call "CRYStep Write.vi"("StepIdentifier"="", "Default"=FALSE, "Proper VI No"=w823, "Category Name"="Stimulus" ("Step File Name"), "Step File Path"=w815, "Step flattened"=w820, "Step File Name"="Stimulus") -> ()  [unwired: 1 in, 4 out]
      }
      event "Load...": Value Change {
        n169 = event-data() -> ("CtlRef"=w824:refnum<vi>)  [unwired: 6 out]
        n170 = local read "Load Test"() -> (w826:bool)
        n171 = property class="Bool (strict)"(reference=w824, "Value"=FALSE) -> ()  [unwired: 1 in, 2 out]
        n172 = case shown="False" w826 {
          frame False {
            n173 = global read "CRYMainGlobal.vi" "Steps path"() -> (w834:path)
            n174 = local read "Proper VI No"() -> (w827:i32)
            n175 = Build Path(base path=w834, name or relative path="CRYStimulus") -> (appended path=w833:path)
            n176 = call "CRYStep Read.vi"("Category Name"="Stimulus", "Proper VI No"=w827, "Step File Path"=w833) -> ("status"=w830:bool, "selected path"=w828:path, "Flatten Step"=w829:string)  [unwired: 1 in, 3 out]
            n177 = case shown="True" w830 {
              tunnel: w829 -> [_ w836]
              tunnel: w828 -> [_ w835]
              tunnel: w827 -> [_ w837]
              frame False {
              }
              frame True {
                n178 = call "CRYUnflatten Stimulus.vi"("Flatten Stimulus"=w836) -> ("Error?"=w838:bool, "Stimulus"=w839:T1)  [unwired: 9 out]
                n179 = case shown="False" w838 {
                  tunnel: w839 -> [w843 _]
                  tunnel: w837 -> [w842 _]
                  tunnel: w836 -> [w841 _]
                  tunnel: w835 -> [w840 _]
                  frame False {
                    n180 = flat-sequence {
                      tunnel: w843 -> [w855]
                      tunnel: w842 -> [w851]
                      tunnel: w841 -> [w850]
                      tunnel: w840 -> [w849]
                      frame #0 {
                        n181 = Strip Path(path=w849) -> (name=w845:string)  [unwired: 1 out]
                        n182 = Reverse String(1:w845) -> (0:w847:string)
                        n183 = Match Pattern(string=w847, regular expression="[.]") -> (after substring=w848:string)  [unwired: 4 out]
                        n184 = Reverse String(1:w848) -> (0:w844:string)
                        n185 = call "CRYPreUpdate Sequence.vi"("EventName"="Load", "StepName Arg3"=w844, "Proper VI No"=w851, "Project View Step Name Identifier Arg1"="", "Step flattened Arg2"=w850, "AllChangeFlg"=TRUE ("Name/Identifier")) -> ()  [unwired: 10 in]
                        n186 = local write "Stimulus"(w855) -> ()
                      }
                      frame #1 {
                        n187 = local write "Load Test"(TRUE ("Load Test")) -> ()
                      }
                      frame #2 {
                        n188 = disable-structure shown="Disabled" {
                          frame Disabled {
                            n189 = local read "Stimulus"() -> (w857:T1)
                            n190 = property on="Stimulus" class="Clust (strict)"("Val(Sgnl)"=w857) -> ()  [unwired: 2 in, 2 out]
                          }
                          frame Enabled {
                          }
                        }
                      }
                    }
                  }
                  frame True {
                  }
                }
              }
            }
          }
          frame True {
          }
        }
      }
      event "Revert": Value Change {
        n191 = event-data() -> ("CtlRef"=w859:refnum<vi>)  [unwired: 6 out]
        n192 = property class="Bool (strict)"(reference=w859, "Value"=FALSE) -> ()  [unwired: 1 in, 2 out]
        n193 = flat-sequence {
          frame #0 {
            n194 = local read "Stimulus Bk"() -> (w860:T1)
            n195 = local write "Stimulus"(w860) -> ()
          }
          frame #1 {
            n196 = local write "Load Test"(TRUE ("Load Test")) -> ()
          }
        }
      }
      event Panel Close {
        n197 = event-data() -> ()  [unwired: 5 out]
        n198 = control-ref of="This VI"() -> (w863:refnum<vi>)
        n199 = local write "Cancel"(TRUE ("Cancel")) -> ()
        n200 = call "CRYWork Before Step Close.vi"("StepVI Ref"=w863) -> ()  [unwired: 11 in]
      }
      event "CurLibChange": Value Change {
        n201 = event-data() -> ()  [unwired: 7 out]
        n202 = global read "CRYRef nums global.vi" "Stimulus Sub VI ref"() -> (w867:refnum<vi>)
        n203 = call "CRYGet Boolean Reference.vi"("Label Name"="CurLibChange", "VI Refnum"=w867) -> ("Exist?"=w865:bool, "Boolean Ref"=w864:refnum<vi>)  [unwired: 7 in, 1 out]
        n204 = case shown="True" w865 {
          tunnel: w864 -> [_ w869]
          frame False {
          }
          frame True {
            n205 = property class="Bool"(reference=w869, "Val(Sgnl)"=TRUE) -> ()  [unwired: 1 in, 2 out]
          }
        }
      }
      event "Help": Value Change {
        n206 = event-data() -> ("NewVal"=w871:string)  [unwired: 6 out]
        n207 = local read "Stimulus"() -> (w872:T1)
        n208 = Bundle By Name(cluster=w872, "Help"=w871) -> (w870:T1)
        n209 = local write "Stimulus"(w870) -> ()
      }
      event "Help Change": Value Change {
        n210 = event-data() -> ("NewVal"=w874:string)  [unwired: 6 out]
        n211 = local read "Stimulus"() -> (w875:T1)
        n212 = Bundle By Name(cluster=w875, "Help"=w874) -> (w873:T1)
        n213 = property on="Help" class="Str"("Val(Sgnl)"=w874) -> ()  [unwired: 2 in, 2 out]
        n214 = local write "Stimulus"(w873) -> ()
      }
      event "Multicolumn Listbox": Double Click {
        n215 = event-data() -> ()  [unwired: 10 out]
        n216 = local write "Edit"(TRUE ("Value (Signaling)")) -> ()
      }
      event "Flatten Element Array": Value Change {
        n217 = event-data() -> ()  [unwired: 7 out]
        n218 = local read "Flatten Element Array"() -> (w878:string[])
        n219 = local read "Stimulus"() -> (w879:T1)
        n220 = Bundle By Name(cluster=w879, "Flatten Element Array"=w878) -> (w877:T1)
        n221 = local write "Stimulus"(w877) -> ()
      }
      event "Custom Stimulus Name": Value Change {
        n222 = event-data() -> ("NewVal"=w884:string)  [unwired: 6 out]
        n223 = local read "Stimulus"() -> (w886:T1)
        n224 = Unbundle By Name(w886) -> ("CustomStimulusName"=w882:string)
        n225 = Bundle By Name(cluster=w886, "CustomStimulusName"=w884) -> (w880:T1)
        n226 = call <vilib>:"Trim Whitespace.vi"("string"=w884) -> ("trimmed string"=w883:string)  [unwired: 1 in]
        n227 = call <vilib>:"Trim Whitespace.vi"("string"=w882) -> ("trimmed string"=w881:string)  [unwired: 1 in]
        n228 = local write "Stimulus"(w880) -> ()
        n229 = Not Equal?(x=w881, y=w883) -> (x != y?=w885:bool)
        n230 = local write "Is Change?"(w885) -> ()
      }
      event "Apply EQ": Value Change {
        n231 = event-data() -> ("NewVal"=w889:bool)  [unwired: 6 out]
        n232 = local read "Stimulus"() -> (w891:T1)
        n233 = Unbundle By Name(w891) -> ("ApplyEQ"=w890:bool)
        n234 = Not Equal?(x=w890, y=w889) -> (x != y?=w888:bool)
        n235 = local write "Is Change?"(w888) -> ()
        n236 = Bundle By Name(cluster=w891, "ApplyEQ"=w889) -> (w887:T1)
        n237 = local write "Stimulus"(w887) -> ()
      }
      event Scale Range Change; Autoscale Range Change; Value Change; Plot Attribute Change {
        n238 = event-data() -> ()  [unwired: 5 out]
        n239 = control-ref of="Wave graph"() -> (w893:refnum<vi>)
        n240 = call "CRYPaint WaterMark.vi"("Type"="Small", "Graph Ref"=w893) -> ()  [unwired: 10 in]
      }
    }
    n241 = Unbundle By Name(w75) -> ("start"=w73:bool)
    n242 = control-ref of="Multicolumn Listbox"() -> (w58:refnum<vi>)
    n243 = property class="MCListbox (strict)"(reference=w58) -> (reference out=w56:refnum<vi>, "Value"=w57:i32)  [unwired: 1 in, 1 out]
    n244 = Compound Arithmetic op=AND(w73, invert "Play") -> (w50:bool)
    n245 = Compound Arithmetic op=AND(invert w73, "Play") -> (w49:bool)
    n246 = Compound Arithmetic op=OR(w49, w50, "Play") -> (w74:bool)
    n247 = Bundle("Load Test"="Load Test", "Output Channel"="Output Channel", "Edit"="Edit", "Insert"="Insert", "Remove"="Remove", "Move Up"="Move Up", "Move Down"="Move Down", "ViewTable"="ViewTable", "View Edit"="View Edit", "Add Lib"="Add Lib", "OK"="OK", "Cancel"="Cancel") -> (w80:T16)  [unwired: 1 out]
    n248 = Quotient & Remainder(x=w57, y=2) -> (floor(x/y)=w55:i32)  [unwired: 1 out]
    n249 = Cluster To Array(cluster=w80) -> (array=w79:bool[])
    n250 = case shown="True" w74 {
      tunnel: w75 -> [w90 w96]
      tunnel: [w90 w98] -> w45
      tunnel: w50 -> [_ w97]
      tunnel: w49 -> [_ w95]
      frame False {
      }
      frame True {
        n251 = local read "Sens Value"() -> (w92:dbl)
        n252 = local read "Vp Out"() -> (w93:dbl)
        n253 = local read "Stim max value"() -> (w94:sgl)
        n254 = call "CRYCheck Amplitude.vi"("Sens Value"=w92, "Vp Out"=w93, "Stimulus max value"=w94) -> ("Overflow"=w91:bool)  [unwired: 8 in]
        n255 = case shown="False" w91 {
          tunnel: [w129 w208] -> w98
          tunnel: w97 -> [w128 _]
          tunnel: w96 -> [w125 w209]
          tunnel: w95 -> [w118 _]
          frame False {
            n256 = case shown="True" w118 {
              tunnel: [w185 w186] -> w103
              frame False {
                n257 = local read "Stimulus Play Wave"() -> (w185:sgl[])
              }
              frame True {
                n258 = stacked-sequence {
                  tunnel: [_ w188] -> w186
                  frame #0 {
                    n259 = local read "Stimulus Wave"() -> (→"Stimulus Play Wave":sgl[])
                  }
                  frame #1 {
                    n260 = local read "Stimulus Play Wave"() -> (w188:sgl[])
                  }
                }
              }
            }
            n261 = Array Size(array=w103) -> (size(s)=w114:i32)
            n262 = local read "Channel Out"() -> (w109:u32)
            n263 = local read "BitDepth"() -> (w110:u32)
            n264 = local read "Asio Inited"() -> (w106:bool)
            n265 = local read "Output Device"() -> (w112:i16)
            n266 = local read "Device Name"() -> (w107:string)
            n267 = local read "Audio Driver"() -> (w105:u16)
            n268 = Not(x=w128) -> (.not. x?=w127:bool)
            n269 = local read "Buffer Index"() -> (w104:u32)
            n270 = local read "Fs"() -> (w111:u32)
            n271 = Multiply(x=w111, y=0.5) -> (x*y=w115:dbl)
            n272 = Subtract(x=w115, y=w114) -> (x-y=w113:dbl)
            n273 = Greater Than 0?(x=w113) -> (x > 0?=w117:bool)
            n274 = case shown="True" w117 {
              tunnel: w103 -> [w179 w184]
              tunnel: w113 -> [_ w183]
              tunnel: [w179 w180] -> w108
              frame False {
              }
              frame True {
                n275 = Initialize Array(sgl 0.0, w183) -> (w181:sgl[])
                n276 = Build Array (concatenate)(w184, w181) -> (w180:sgl[])
              }
            }
            n277 = Divide(x=w114, y=w111) -> (x/y=w124:dbl)
            n278 = Interleave 1D Arrays(w108, w108) -> (w120:sgl[])
            n279 = Array Size(array=w120) -> (size(s)=w119:i32)
            n280 = To Unsigned Long Integer(number=w119) -> (unsigned 32bit integer=w123:u32)
            n281 = Boolean To (0,1)(Boolean=w127) -> (0, 1=w126:i16)
            n282 = Multiply(x=u32 4, y=w123) -> (x*y=w122:u32)
            n283 = case shown="2" w105 {
              tunnel: w126 -> [_ w178]
              tunnel: [w138 w168] -> w102
              tunnel: w124 -> [_ w167]
              tunnel: w122 -> [_ w166]
              tunnel: w120 -> [_ w163]
              tunnel: w112 -> [_ w162]
              tunnel: w111 -> [w141 w161]
              tunnel: w110 -> [w139 w160]
              tunnel: w109 -> [w140 w159]
              tunnel: w108 -> [w130 _]
              tunnel: w107 -> [w142 _]
              tunnel: w106 -> [w137 _]
              tunnel: w104 -> [w136 _]
              frame 2 {
                w132 = 4194303.0  # 2^22 - 1
                n284 = case shown="False" w137 {
                  tunnel: w140 -> [w157 _]
                  tunnel: w142 -> [w156 _]
                  tunnel: w141 -> [w155 _]
                  tunnel: w139 -> [w154 _]
                  tunnel: [w153 w158] -> w143
                  frame False {
                    n285 = local write "Buffer Index"(u32 0 ("Buffer Index")) -> ()
                    n286 = call "CRYASIO Out & Init & Start.vi"("Bit Depth"=w154, "Sampling Rate"=w155, "Channel Index"=w157, "Device Name"=w156) -> ("bResult"=w151:bool, "Asio Opend Channel Index"=w153:u32)  [unwired: 6 in]
                    n287 = local write "Asio Inited"(w151) -> ()
                    n288 = local write "Asio Limit"(w153) -> ()
                  }
                  frame True {
                    n289 = local read "Asio Limit"() -> (w158:u32)
                  }
                }
                n290 = call "CRYMake Asio Buffer.vi"("Fs"=u32 0, "Buffer Index"=w136, "Data Array"=w130) -> ("BufferIsEmpty?"=w138:bool, "Buf Data"=w131:sgl[])  [unwired: 7 in]
                n291 = local read "Asio Inited"() -> (w135:bool)
                n292 = Divide(x=w131, y=w132) -> (x/y=w133:dbl[])
                n293 = To Single Precision Float(number=w133) -> (single precision float=w134:sgl[])
                n294 = case shown="True" w135 {
                  tunnel: w134 -> [_ w150]
                  tunnel: w143 -> [_ w149]
                  frame False {
                  }
                  frame True {
                    n295 = local read "Buffer Index"() -> (w146:u32)
                    n296 = local read "Buf Amount"() -> (w147:u32)
                    n297 = call "CRYASIO Play Buffer Stimulus.vi"("Data Array"=w150, "Buffer Index"=w146, "Buffer Amount"=w147, "Limit"=w149) -> ("Buffer Index Out"=w145:u32, "Buffer Amount Out"=w148:u32)  [unwired: 5 in]
                    n298 = local write "Buffer Index"(w145) -> ()
                    n299 = local write "Buf Amount"(w148) -> ()
                  }
                }
              }
              frame 0, Default {
                w165 = u8 0 ("pauseflag")
                n300 = local read "ntaskID"() -> (w169:u32)
                n301 = dll-call lib="D:/A_CRYSoundLab_Work/CRY6181/CRYSound.dll" fn="GVPlayMemory"("DeviceID"=w162, "pSampleData"=w163, "InSampleFreq"=w161, "nInbitDepth"=u32 32, "nInChannels"=u32 2, "nInSampleLen"=w166, "OutSampleFreq"=w161, "nOutbitDepth"=w160, "nOutChannels"=w159, "PlayMode"=u32 2, "Duration"=w167, "nTimes"=u32 1, "OutLevel"=1.0 ("x/y"), "startflag"=w178, "pauseflag"=w165, "changeflag"=w165, "ntaskID"=w169) -> ("return type"=w176:u32, "ntaskID"=w170:u32)  [unwired: 17 in, 4 out]
                n302 = local write "ntaskID"(w170) -> ()
                n303 = Not Equal?(x=w176, y=u32 0) -> (x != y?=w168:bool)
                n304 = Less Or Equal?(x=w176, y=u32 1) -> ()  [unwired: 1 out]
              }
            }
            n305 = local read "Play"() -> (w100:bool)
            n306 = Not(x=w100) -> (.not. x?=w99:bool)
            n307 = Or(x=w102, y=w99) -> (x .or. y?=w101:bool)
            n308 = case shown="True" w101 {
              tunnel: w125 -> [w190 w196]
              tunnel: [w189 w195] -> w129
              tunnel: w105 -> [_ w193]
              frame False {
                n309 = Bundle By Name(cluster=w190, "start"=TRUE) -> (w189:T5)
              }
              frame True {
                w194 = FALSE ("start")
                n310 = Bundle By Name(cluster=w196, "start"=w194) -> (w195:T5)
                n311 = local write "Play"(w194) -> ()
                n312 = local read "Asio Inited"() -> (w192:bool)
                n313 = case shown="2" w193 {
                  tunnel: w192 -> [_ w197]
                  frame 0, Default {
                  }
                  frame 2 {
                    n314 = case shown="True" w197 {
                      frame False {
                      }
                      frame True {
                        n315 = flat-sequence {
                          frame #0 {
                            n316 = local read "Buf Amount"() -> (w202:u32)
                            n317 = local read "Fs"() -> (w201:u32)
                            n318 = Divide(x=w202, y=w201) -> (x/y=w200:dbl)
                            n319 = Multiply(x=w200, y=1000.0) -> (x*y=w199:dbl)
                            n320 = Wait (ms)(milliseconds to wait=w199) -> ()  [unwired: 1 out]
                          }
                          frame #1 {
                            n321 = local read "Asio Limit"() -> (w204:u32)
                            n322 = local read "Channel Out"() -> (w203:u32)
                            n323 = local write "Buffer Index"(u32 0 ("Buffer Index")) -> ()
                            n324 = local write "Asio Inited"(FALSE ("Asio Inited")) -> ()
                            n325 = call "CRYASIO Close Cur Channel & Dev.vi"("Limit"=w204, "isInput?"=FALSE, "Channel Out"=w203) -> ()  [unwired: 9 in]
                          }
                        }
                      }
                    }
                  }
                }
              }
            }
          }
          frame True {
            w210 = FALSE ("start")
            n326 = call "CRYGet Error Message.vi"("Error No"=9, "Kind"="Stimulus") -> ("Message"=w212:string, "Window Title"=w211:string)  [unwired: 4 in, 4 out]
            n327 = call "CRYMessage Dialog.vi"("Window Title"=w211, "Message Content"=w212) -> ()  [unwired: 8 in, 2 out]
            n328 = Bundle By Name(cluster=w209, "start"=w210) -> (w208:T5)
            n329 = local write "Play"(w210) -> ()
          }
        }
      }
    }
    n330 = Search 1D Array(1D array=w79, element=TRUE) -> (index of element=w77:i32)  [unwired: 1 out]
    n331 = case shown="9" w77 {
      tunnel: w57 -> [_ _ _ w374 w414 _ _ _ _ _ _ _ _]
      tunnel: w56 -> [_ _ _ w372 w416 _ _ _ _ _ _ _ _]
      tunnel: w55 -> [_ _ _ w371 w411 _ _ _ _ _ _ _ _]
      tunnel: w53 -> [_ w216 _ _ _ _ _ _ _ _ _ _ _]
      tunnel: w52 -> [_ w215 _ _ _ _ _ _ _ _ _ _ _]
      frame Default {
      }
      frame 0 {
        n332 = stacked-sequence {
          tunnel: w216 -> [w240 _ _]
          tunnel: w215 -> [w239 _ _]
          frame #0 {
            # "????"
            n333 = local read "Stimulus"() -> (w252:T1)
            n334 = local read "Calibration setup In"() -> (w225:string)
            n335 = Unbundle By Name(w252) -> ("Duration(s)"=w250:dbl, "CustomStimulusName"=w247:string, "ApplyEQ"=w251:bool, "Flatten Element Array"=w249:string[], "Signal Type Name"=w226:string, "Channel Out"=w241:i32)
            n336 = local write "Is Change?"(TRUE ("Is Change?")) -> ()
            n337 = call "CRYUnflatten Calibration 2D.vi"("Flattened Calibration"=w225) -> ("Calibration Step Out"=w224:T7)  [unwired: 8 in, 2 out]
            n338 = property on="Apply EQ" class="Bool (strict)"("Value"=w251) -> ()  [unwired: 2 in, 2 out]
            n339 = property on="Flatten Element Array" class="Arr (strict)"("Value"=w249) -> ()  [unwired: 2 in, 2 out]
            n340 = property on="Duration(s)" class="DigNum (strict)"("Value"=w250) -> ()  [unwired: 2 in, 2 out]
            n341 = call "CRYGet Cal Info From SignalType and Channel Name.vi"("Calibration"=w224, "Signal Type"=w226, "In/Out?"=FALSE) -> ("Calibration 2D Cluster"=w223:T8)  [unwired: 6 in, 2 out]
            n342 = Unbundle By Name(w223) -> ("Calibration.Cha Name"=w222:string)
            n343 = call "CRYGet Current TS Steps.vi"() -> ("SelectStepNumber in Tree"=w219:i32, "Steps"=w220:T11[])  [unwired: 1 in, 9 out]
            n344 = call "CRYCheck Channel Info.vi"("Is Input?"=FALSE, "Channel No"=w241, "Channel Name"=w222) -> ("Channel Info"=w234:T2, "ID"=w235:i32, "Is exist?"=w242:bool)  [unwired: 6 out]
            n345 = Index Array(array=w220, index=w219) -> (element=w218:T11)
            n346 = case shown="True" w242 {
              tunnel: w226 -> [_ w258]
              tunnel: w241 -> [_ _]
              tunnel: [w254 w258] -> w238
              tunnel: [w255 w260] -> w237
              tunnel: w240 -> [w254 _]
              tunnel: w239 -> [w255 _]
              tunnel: w235 -> [_ _]
              tunnel: w234 -> [_ w264]
              tunnel: w226 -> [_ _]
              frame False {
              }
              frame True {
                n347 = Unbundle By Name(w264) -> ("Audio Driver"=w257:u16, "Device Name"=w256:string, "Hardware Ch ID"=w260:u8, "ID"=w259:i32, "Sampling Rate (Hz)"=w263:u32, "Bit Depth"=w262:u32, "Vmax (V)"=w261:dbl)
                n348 = local write "Audio Driver"(w257) -> ()
                n349 = local write "Device Name"(w256) -> ()
                n350 = local write "Output Device"(w259) -> ()
                n351 = local write "BitDepth"(w262) -> ()
                n352 = local write "Vp Out"(w261) -> ()
                n353 = local write "Fs"(w263) -> ()
              }
            }
            n354 = Unbundle By Name(w218) -> ("StepName"=w217:string)
            n355 = Equal?(x=w247, y="") -> (x = y?=w248:bool)
            n356 = Select(t=w217, s=w248, f=w247) -> (s? t:f=w244:string)
            n357 = local write "Signal Type Name"(w238) -> ()
            n358 = local write "Channel Out"(w237) -> ()
            n359 = local read "O_channel Info Out"() -> (w233:T2[])
            n360 = property on="Custom Stimulus Name" class="Str"("Value"=w244) -> ()  [unwired: 2 in, 2 out]
            n361 = Array Size(array=w233) -> (size(s)=w232:i32)
            n362 = Greater Than 0?(x=w232) -> (x > 0?=w231:bool)
            n363 = local read "Stimulus"() -> (w245:T1)
            n364 = Bundle By Name(cluster=w245, "CustomStimulusName"=w244, "Signal Type Name"=w238, "Channel Out"=w237) -> (w221:T1)
            n365 = Select(t=T12."Enabled" ("Disabled"), s=w231, f=T12."Disabled and Grayed Out" ("Disabled")) -> (s? t:f=w229:T12)
            n366 = property on="Output Channel" class="Bool"("DisabledEnum"=w229) -> ()  [unwired: 2 in, 2 out]
            n367 = property on="Play" class="Bool (strict)"("DisabledEnum"=w229) -> ()  [unwired: 2 in, 2 out]
            n368 = disable-structure shown="Disabled" {
              disable-tunnel: w221 -> [w253 _]
              frame Disabled {
                n369 = property on="Stimulus" class="Clust (strict)"("Val(Sgnl)"=w253) -> ()  [unwired: 2 in, 2 out]
              }
              frame Enabled {
              }
            }
            n370 = property on="Stimulus" class="Clust (strict)"("Value"=w221) -> ()  [unwired: 2 in, 2 out]
          }
          frame #1 {
            n371 = local read "Flatten Element Array"() -> (w265:string[])
            n372 = Index Array(array=w265) -> (element=w266:string)  [unwired: 1 in]
            n373 = global write "CRYStimulus Global.vi" "Flatten Element"(w266) -> ()
            n374 = Array Size(array=w265) -> (size(s)=w269:i32)
            n375 = Greater?(x=w269, y=1) -> (0:w267:bool)
            n376 = case shown="True" w267 {
              tunnel: w265 -> [_ w285]
              frame False {
                n377 = stacked-sequence {
                  frame #0 {
                    n378 = local read "Stimulus"() -> (w270:T1)
                    n379 = global write "CRYStimulus Global.vi" "Stimulus Cluster"(w270) -> ()
                  }
                  frame #1 {
                    n380 = property on="Is SubPan?" class="Bool (strict)"() -> ("Value"=w271:bool)  [unwired: 2 in, 2 out]
                    n381 = case shown="False" w271 {
                      frame False {
                        n382 = flat-sequence {
                          frame #0 {
                            w272 = FALSE ("Visible")
                            n383 = property on="Table Tab" class="TabCtl (strict)"("Visible"=w272) -> ()  [unwired: 2 in, 2 out]
                            n384 = property on="ViewTable" class="Bool"("Visible"=TRUE) -> ()  [unwired: 2 in, 2 out]
                            n385 = property on="Is SubPan?" class="Bool (strict)"("Value"=TRUE ("Is SubPan?")) -> ()  [unwired: 2 in, 2 out]
                            n386 = property on="View Edit" class="Bool"("Visible"=w272) -> ()  [unwired: 2 in, 2 out]
                          }
                          frame #1 {
                            n387 = global read "CRYRef nums global.vi" "Stimulus Sub VI ref"() -> (w275:refnum<vi>)
                            n388 = property class="VI"(reference=w275, "FP.Behavior"=T13."Default" ("Front Panel Window:Behavior")) -> (reference out=w279:refnum<vi>)  [unwired: 1 in, 1 out]
                            n389 = invoke class="VI" method="Run VI"(reference=w279, "Wait until done"=FALSE ("Wait Until Done")) -> (reference out=w277:refnum<vi>)  [unwired: 3 in, 4 out]
                            n390 = local write "reference out"(w277) -> ()
                            n391 = invoke on="Sub Panel" class="SubPanel" method="Insert VI"("VI Ref"=w277) -> ()  [unwired: 3 in, 4 out]
                          }
                        }
                      }
                      frame True {
                      }
                    }
                  }
                  frame #2 {
                    n392 = local read "reference out"() -> (w281:refnum<vi>)
                    n393 = local read "Stimulus"() -> (w282:T1)
                    n394 = call "CRYGet String Reference.vi"("Label Name"="Stimulus Change", "VI Refnum"=w281) -> ("String Ref Out"=w284:refnum<vi>)  [unwired: 9 out]
                    n395 = call "CRYFlatten Stimulus.vi"("Stimulus"=w282) -> ("Flatten Stimulus String"=w283:string)  [unwired: 10 out]
                    n396 = property class="Str"(reference=w284, "Val(Sgnl)"=w283) -> ()  [unwired: 1 in, 2 out]
                  }
                }
              }
              frame True {
                n397 = flat-sequence {
                  tunnel: [w288] -> w286
                  tunnel: w285 -> [w288]
                  tunnel: w286 -> [w294]
                  frame #0 {
                    n398 = property on="Is SubPan?" class="Bool (strict)"() -> ("Value"=w287:bool)  [unwired: 2 in, 2 out]
                    n399 = case shown="True" w287 {
                      frame False {
                      }
                      frame True {
                        n400 = flat-sequence {
                          frame #0 {
                            n401 = invoke on="Sub Panel" class="SubPnl" method="Remove VI"() -> ()  [unwired: 3 in, 3 out]
                          }
                          frame #1 {
                            n402 = local read "reference out"() -> (w290:refnum<vi>)
                            n403 = call "CRYGet Boolean Reference.vi"("Label Name"="stop", "VI Refnum"=w290) -> ("Boolean Ref"=w292:refnum<vi>)  [unwired: 7 in, 2 out]
                            n404 = property class="Bool"(reference=w292, "Val(Sgnl)"=TRUE ("Front Panel.Open")) -> ()  [unwired: 1 in, 2 out]
                          }
                        }
                      }
                    }
                    n405 = property on="Multicolumn Listbox" class="MCListbox (strict)"("ItemNames"=string[][] [] ("Item Names")) -> ()  [unwired: 2 in, 2 out]
                  }
                  frame #1 {
                    n406 = for {
                      tunnel: w294 -> [w297] mode=indexing
                      n407 = control-ref of="Multicolumn Listbox"() -> (w296:refnum<vi>)
                      n408 = call "CRYStimulus Table Insert.vi"("Insert"=TRUE, "Stimulus TableRef"=w296, "Flatten Stimulus Setup String"=w297) -> ()  [unwired: 9 out]
                    }
                  }
                  frame #2 {
                    n409 = property on="Remove" class="Bool"("DisabledEnum"=T12."Enabled" ("Disabled")) -> ()  [unwired: 2 in, 2 out]
                    n410 = property on="Table Tab" class="TabCtl (strict)"("Visible"=TRUE) -> ()  [unwired: 2 in, 2 out]
                    n411 = property on="Is SubPan?" class="Bool (strict)"("Value"=FALSE ("Is SubPan?")) -> ()  [unwired: 2 in, 2 out]
                    n412 = property on="ViewTable" class="Bool"("Visible"=FALSE) -> ()  [unwired: 2 in, 2 out]
                    n413 = property on="View Edit" class="Bool"("Visible"=TRUE, "DisabledEnum"=T12."Disabled and Grayed Out" ("Disabled")) -> ()  [unwired: 2 in, 2 out]
                  }
                }
              }
            }
          }
          frame #2 {
            n414 = flat-sequence {
              frame #0 {
                w304 = TRUE ("Input/Output")
                n415 = control-ref of="Board Tab"() -> (w306:refnum<vi>)
                n416 = control-ref of="This VI"() -> (w305:refnum<vi>)
                n417 = call "CRYAlign Steps VI Center.vi"("Tab2"=w306, "Input/Output"=w304, "VIRef"=w305) -> ()  [unwired: 1 in, 8 out]
                n418 = property on="Update" class="Bool (strict)"("Val(Sgnl)"=w304) -> ()  [unwired: 2 in, 2 out]
              }
              frame #1 {
                n419 = local write "Load Test"(FALSE ("Load Test")) -> ()
                n420 = property on="Board Tab" class="TabCtl (strict)"("Visible"=TRUE) -> ()  [unwired: 2 in, 2 out]
              }
            }
          }
        }
      }
      frame 1 {
        n421 = local read "Signal Type Name"() -> (w309:string)
        n422 = local read "Calibration setup In"() -> (w314:string)
        n423 = call "CRYGet Current Calibration Info.vi"("Is Input?"=FALSE, "Signal Type Name"=w309) -> ("Calibration All Cluster"=w325:T8)  [unwired: 9 out]
        n424 = Unbundle By Name(w325) -> ("Sens Curve"=w323:T10)
        n425 = Unbundle By Name(w323) -> ("Curve"=w322:cluster{"x":dbl, "y":dbl, "z":dbl}[], "Y dB ref"=w328:dbl, "Y data"=w326:u16)
        n426 = call "CRYUnflatten Calibration 2D.vi"("Flattened Calibration"=w314) -> ("Calibration Step Out"=w317:T7)  [unwired: 8 in, 2 out]
        n427 = property on="O_channel Info Out" class="Arr (strict)"() -> ("Value"=w316:T2[])  [unwired: 2 in, 2 out]
        n428 = Index Array(array=w322) -> (element=w321:cluster{"x":dbl, "y":dbl, "z":dbl})  [unwired: 1 in]
        n429 = Build Array(w309) -> (w315:string[])
        n430 = Unbundle By Name(w321) -> ("y"=w327:dbl)
        n431 = call "CRYSelect Signal Type Dialog.vi"("Channel Info In"=w316, "Selected Signal Type In"=w315, "Mode(0ne or More)"=TRUE, "I/O Calibration In"=w317, "In/Out Signal Type"=FALSE) -> ("Calibration 2D Out"=w310:T8[], "Selected Signal Type"=w313:i32[], "Selected Flag"=w312:bool, "Selected Channel Info Out"=w311:T2[])  [unwired: 3 in]
        n432 = case shown="0, Default" w326 {
          tunnel: w327 -> [w334 w335]
          tunnel: [w333 w335] -> w320
          tunnel: w328 -> [w332 _]
          frame 0, Default {
            n433 = call "CRYConversion dB-Lin.vi"("dB ref."=w332, "Log In"=w334) -> ("Lin Out"=w333:dbl)  [unwired: 4 in, 3 out]
          }
          frame 1 {
          }
        }
        "Sens Value" <- w320
        n434 = Array Size(array=w313) -> (size(s)=w331:i32)
        n435 = Greater Than 0?(x=w331) -> (x > 0?=w330:bool)
        n436 = And(x=w312, y=w330) -> (x .and. y?=w329:bool)
        n437 = case shown="True" w329 {
          tunnel: w311 -> [_ w350]
          tunnel: w309 -> [_ w345]
          tunnel: w310 -> [_ w341]
          frame False {
          }
          frame True {
            n438 = Index Array(array=w341) -> (element=w340:T8)  [unwired: 1 in]
            n439 = Index Array(array=w350, index=0) -> (element=w351:T2)
            n440 = property on="Is SubPan?" class="Bool (strict)"() -> ("Value"=w347:bool)  [unwired: 2 in, 2 out]
            n441 = Unbundle By Name(w340) -> ("Calibration.Signal Type"=w339:string)
            n442 = Not Equal?(x=w339, y=w345) -> (x != y?=w344:bool)
            n443 = Unbundle By Name(w351) -> ("ID"=w353:i32, "Hardware Ch ID"=w346:u8, "Sampling Rate (Hz)"=w343:u32, "Bit Depth"=w352:u32, "Vmax (V)"=w349:dbl, "Audio Driver"=w336:u16, "Device Name"=w337:string)
            n444 = local write "Is Change?"(w344) -> ()
            n445 = case shown="True" w347 {
              tunnel: w349 -> [_ w357]
              tunnel: w339 -> [_ w356]
              tunnel: w343 -> [_ w355]
              frame False {
              }
              frame True {
                n446 = local read "reference out"() -> (w358:refnum<vi>)
                n447 = stacked-sequence {
                  tunnel: w358 -> [w360 w363 w370]
                  tunnel: w356 -> [_ _ w367]
                  tunnel: w357 -> [w359 _ _]
                  tunnel: w355 -> [_ w364 _]
                  frame #0 {
                    n448 = call "CRYGet Numeric Reference.vi"("Label Name"="Vmax (V)", "VI Refnum"=w360) -> ("Numeric Ref Out"=w362:refnum<vi>)  [unwired: 9 out]
                    n449 = property class="DigNum"(reference=w362, "Val(Sgnl)"=w359) -> ()  [unwired: 1 in, 2 out]
                  }
                  frame #1 {
                    n450 = call "CRYGet Numeric Reference.vi"("Label Name"="Sampling Rate (Hz)", "VI Refnum"=w363) -> ("Numeric Ref Out"=w366:refnum<vi>)  [unwired: 9 out]
                    n451 = property class="DigNum"(reference=w366, "Val(Sgnl)"=w364) -> ()  [unwired: 1 in, 2 out]
                  }
                  frame #2 {
                    n452 = call "CRYGet String Reference.vi"("Label Name"="Channel Change", "VI Refnum"=w370) -> ("String Ref Out"=w368:refnum<vi>)  [unwired: 9 out]
                    n453 = property class="Str"(reference=w368, "Val(Sgnl)"=w367) -> ()  [unwired: 1 in, 2 out]
                  }
                }
              }
            }
            n454 = local write "Signal Type Name"(w339) -> ()
            n455 = local write "Output Device"(w353) -> ()
            n456 = local write "Channel Out"(w346) -> ()
            n457 = local write "BitDepth"(w352) -> ()
            n458 = local write "Vp Out"(w349) -> ()
            n459 = local write "Fs"(w343) -> ()
            n460 = local write "Audio Driver"(w336) -> ()
            n461 = local write "Device Name"(w337) -> ()
            n462 = local read "Stimulus"() -> (w348:T1)
            n463 = Bundle By Name(cluster=w348, "Signal Type Name"=w339, "Channel Out"=w346) -> (w338:T1)
            n464 = disable-structure shown="Disabled" {
              disable-tunnel: w338 -> [w354 _]
              frame Disabled {
                n465 = property on="Stimulus" class="Clust (strict)"("Val(Sgnl)"=w354) -> ()  [unwired: 2 in, 2 out]
              }
              frame Enabled {
              }
            }
            n466 = property on="Stimulus" class="Clust (strict)"("Value"=w338) -> ()  [unwired: 2 in, 2 out]
          }
        }
      }
      frame 2 {
        n467 = property on="Edit" class="Bool (strict)"("Value"=FALSE ("Edit")) -> ()  [unwired: 2 in, 2 out]
        n468 = Greater Than 0?(x=w374) -> (x > 0?=w373:bool)
        n469 = case shown="True" w373 {
          tunnel: w372 -> [w381 _]
          tunnel: w371 -> [w376 _]
          frame True {
            n470 = local read "Stimulus"() -> (w380:T1)
            n471 = call "CRYOpen Edit Dialog.vi"("List Index"=w376, "Stimulus In"=w380) -> ("Ok Boolean"=w377:bool, "Flatten Element Out"=w378:string, "Stimulus Out"=w379:T1)  [unwired: 7 out]
            n472 = case shown="True" w377 {
              tunnel: w381 -> [_ w388]
              tunnel: w379 -> [_ w386]
              tunnel: w378 -> [_ w387]
              tunnel: w376 -> [_ w382]
              frame False {
              }
              frame True {
                n473 = flat-sequence {
                  tunnel: w388 -> [w390]
                  tunnel: w387 -> [w391]
                  tunnel: w386 -> [w392]
                  tunnel: [w391] -> w385
                  tunnel: [w390] -> w384
                  tunnel: [w389] -> w383
                  tunnel: w382 -> [w389]
                  tunnel: w385 -> [w395]
                  tunnel: w384 -> [w404]
                  tunnel: w383 -> [w397]
                  frame #0 {
                    n474 = local write "Stimulus"(w392) -> ()
                    n475 = call "CRYStimulus Table Insert.vi"("Insert"=FALSE, "Stimulus TableRef"=w390, "Flatten Stimulus Setup String"=w391) -> ()  [unwired: 9 out]
                  }
                  frame #1 {
                    w399 = FALSE ("display message?")
                    n476 = local read "Flatten Element Array"() -> (w398:string[])
                    n477 = Index Array(array=w398, index=w397) -> (element=w396:string)
                    n478 = call "CRYCheck EditVal.vi"("Is SubPan?"=w399, "display message?"=w399, "MCListbox Refnum"=w404) -> ("Error"=w403:bool)  [unwired: 1 in, 7 out]
                    n479 = call "CRYCheck Change Before Update.vi"("New Flatten Stimulus Element"=w395, "Old Flatten Stimulus Element"=w396) -> ("Is Change?"=w394:bool)  [unwired: 9 out]
                    "Is Change?" <- w394
                    n480 = Not(x=w403) -> (.not. x?=w402:bool)
                    n481 = Not Equal?(x=w395, y="") -> (x != y?=w401:bool)
                    n482 = Compound Arithmetic op=AND(w401, w402, w394) -> (w400:bool)
                    n483 = case shown="True" w400 {
                      tunnel: w395 -> [_ w409]
                      tunnel: w397 -> [_ w408]
                      tunnel: w398 -> [_ w406]
                      frame False {
                      }
                      frame True {
                        n484 = Replace Array Subset(array=w406, new element=w409, index=w408) -> (w407:string[])
                        n485 = property on="Flatten Element Array" class="Arr (strict)"("Val(Sgnl)"=w407) -> ()  [unwired: 2 in, 2 out]
                      }
                    }
                  }
                }
              }
            }
          }
          frame False {
          }
        }
      }
      frame 3 {
        n486 = Less Than 0?(x=w414) -> (x < 0?=w410:bool)
        n487 = Select(t=-1 ("f"), s=w410, f=w411) -> (s? t:f=w413:i32)
        n488 = local read "Stimulus"() -> (w417:T1)
        n489 = call "CRYOpen Edit Dialog.vi"("List Index"=w413, "Stimulus In"=w417) -> ("Ok Boolean"=w415:bool, "Flatten Element Out"=w419:string, "Stimulus Out"=w418:T1)  [unwired: 7 out]
        n490 = case shown="True" w415 {
          tunnel: w419 -> [_ w425]
          tunnel: w418 -> [_ w424]
          tunnel: w416 -> [_ w423]
          tunnel: w413 -> [_ w422]
          tunnel: w410 -> [_ w421]
          frame False {
          }
          frame True {
            n491 = flat-sequence {
              tunnel: w425 -> [w429]
              tunnel: w424 -> [w430]
              tunnel: w423 -> [w428]
              tunnel: [w429] -> w427
              tunnel: [w428] -> w426
              tunnel: w427 -> [w440]
              tunnel: w422 -> [w439]
              tunnel: w426 -> [w437]
              tunnel: w421 -> [w432]
              frame #0 {
                n492 = local write "Stimulus"(w430) -> ()
                n493 = call "CRYStimulus Table Insert.vi"("Insert"=TRUE, "Stimulus TableRef"=w428, "Flatten Stimulus Setup String"=w429) -> ()  [unwired: 9 out]
              }
              frame #1 {
                w433 = FALSE ("display message?")
                n494 = call "CRYCheck EditVal.vi"("Is SubPan?"=w433, "display message?"=w433, "MCListbox Refnum"=w437) -> ("Error"=w438:bool)  [unwired: 1 in, 7 out]
                n495 = Not Equal?(x=w440, y="") -> (x != y?=w435:bool)
                n496 = Not(x=w438) -> (.not. x?=w436:bool)
                n497 = And(x=w435, y=w436) -> (x .and. y?=w434:bool)
                n498 = case shown="True" w434 {
                  tunnel: w440 -> [_ w449]
                  tunnel: w439 -> [_ w448]
                  tunnel: w432 -> [_ w443]
                  frame False {
                  }
                  frame True {
                    n499 = local read "Flatten Element Array"() -> (w447:string[])
                    n500 = Increment(x=w448) -> (x+1=w445:i32)
                    n501 = case shown="False" w443 {
                      tunnel: w449 -> [w453 w455]
                      tunnel: w447 -> [w452 w456]
                      tunnel: [w451 w454] -> w446
                      tunnel: w445 -> [w450 _]
                      frame False {
                        n502 = Insert Into Array(array=w452, index=w450, new element=w453) -> (w451:string[])
                      }
                      frame True {
                        n503 = Insert Into Array(array=w456, new element=w455) -> (w454:string[])  [unwired: 1 in]
                      }
                    }
                    n504 = local write "Is Change?"(TRUE ("Is Change?")) -> ()
                    n505 = property on="Flatten Element Array" class="Arr (strict)"("Val(Sgnl)"=w446) -> ()  [unwired: 2 in, 2 out]
                    n506 = property on="View Edit" class="Bool"("DisabledEnum"=T12."Disabled and Grayed Out" ("Disabled")) -> ()  [unwired: 2 in, 2 out]
                  }
                }
              }
            }
            n507 = property on="Remove" class="Bool"("DisabledEnum"=T12."Enabled" ("Disabled")) -> ()  [unwired: 2 in, 2 out]
          }
        }
      }
      frame 4 {
        n508 = local read "Flatten Element Array"() -> (w462:string[])
        n509 = property on="Multicolumn Listbox" class="MCListbox (strict)"() -> ("Value"=w464:i32)  [unwired: 2 in, 2 out]
        n510 = Greater?(x=w464, y=0) -> (0:w458:bool)
        n511 = Array Size(array=w462) -> (size(s)=w461:i32)
        n512 = Greater?(x=w461, y=1) -> (0:w457:bool)
        n513 = And(x=w458, y=w457) -> (x .and. y?=w459:bool)
        n514 = case shown="True" w459 {
          tunnel: w464 -> [_ w475]
          tunnel: w462 -> [_ w465]
          frame False {
          }
          frame True {
            n515 = property on="Multicolumn Listbox" class="MCListbox (strict)"() -> ("ItemNames"=w474:string[][])  [unwired: 2 in, 2 out]
            n516 = Decrement(x=w475) -> (x-1=w472:i32)
            n517 = Delete From Array(array=w474, index (row)=w472) -> (array with subset deleted=w473:string[][])  [unwired: 2 in, 1 out]
            n518 = Quotient & Remainder(x=w475, y=2) -> (floor(x/y)=w469:i32)  [unwired: 1 out]
            n519 = Delete From Array(array=w473, index (row)=w472) -> (array with subset deleted=w471:string[][])  [unwired: 2 in, 1 out]
            n520 = Delete From Array(array=w465, index=w469) -> (array with subset deleted=w467:string[])  [unwired: 1 in, 1 out]
            n521 = property on="Multicolumn Listbox" class="MCListbox (strict)"("ItemNames"=w471) -> ()  [unwired: 2 in, 2 out]
            n522 = property on="Flatten Element Array" class="Arr (strict)"("Val(Sgnl)"=w467) -> ()  [unwired: 2 in, 2 out]
            n523 = Array Size(array=w467) -> (size(s)=w466:i32)
            n524 = local write "Is Change?"(TRUE ("Is Change?")) -> ()
            n525 = case shown="1" w466 {
              frame Default {
              }
              frame 1 {
                n526 = property on="View Edit" class="Bool"("DisabledEnum"=T12."Enabled" ("Disabled")) -> ()  [unwired: 2 in, 2 out]
                n527 = property on="Remove" class="Bool"("DisabledEnum"=T12."Disabled and Grayed Out" ("Disabled")) -> ()  [unwired: 2 in, 2 out]
              }
            }
          }
        }
      }
      frame 5 {
        n528 = property on="Multicolumn Listbox" class="MCListbox (strict)"() -> ("Value"=w478:i32)  [unwired: 2 in, 2 out]
        n529 = Greater?(x=w478, y=1) -> (0:w480:bool)
        n530 = case shown="True" w480 {
          tunnel: w478 -> [_ w491]
          frame False {
          }
          frame True {
            n531 = property on="Multicolumn Listbox" class="MCListbox (strict)"() -> ("ItemNames"=w500:string[][])  [unwired: 2 in, 2 out]
            n532 = local read "Flatten Element Array"() -> (w483:string[])
            n533 = Subtract(x=w491, y=3) -> (x-y=w489:i32)
            n534 = Decrement(x=w491) -> (x-1=w492:i32)
            n535 = Increment(x=w489) -> (x+1=w484:i32)
            n536 = Delete From Array(array=w500, index (row)=w489) -> (deleted portion=w497:string[], array with subset deleted=w499:string[][])  [unwired: 2 in]
            n537 = Delete From Array(array=w499, index (row)=w489) -> (deleted portion=w495:string[], array with subset deleted=w498:string[][])  [unwired: 2 in]
            n538 = Quotient & Remainder(x=w484, y=2) -> (floor(x/y)=w486:i32)  [unwired: 1 out]
            n539 = Insert Into Array(array=w498, index (row)=w492, new element=w497) -> (w496:string[][])  [unwired: 1 in]
            n540 = Delete From Array(array=w483, index=w486) -> (deleted portion=w487:string, array with subset deleted=w488:string[])  [unwired: 1 in]
            n541 = Insert Into Array(array=w496, index (row)=w491, new element=w495) -> (w494:string[][])  [unwired: 1 in]
            n542 = Increment(x=w486) -> (x+1=w485:i32)
            n543 = property on="Multicolumn Listbox" class="MCListbox (strict)"("ItemNames"=w494) -> ()  [unwired: 2 in, 2 out]
            n544 = Insert Into Array(array=w488, index=w485, new element=w487) -> (w482:string[])
            n545 = property on="Flatten Element Array" class="Arr (strict)"("Val(Sgnl)"=w482) -> ()  [unwired: 2 in, 2 out]
            n546 = property on="Multicolumn Listbox" class="MCListbox (strict)"("Value"=w484) -> ()  [unwired: 2 in, 2 out]
            n547 = local write "Is Change?"(TRUE ("Is Change?")) -> ()
          }
        }
      }
      frame 6 {
        n548 = property on="Multicolumn Listbox" class="MCListbox (strict)"() -> ("ItemNames"=w501:string[][])  [unwired: 2 in, 2 out]
        n549 = Array Size(array=w501) -> (size(s)=w502:i32[])
        n550 = Index Array(array=w502, index=0) -> (element=w504:i32)
        n551 = property on="Multicolumn Listbox" class="MCListbox (strict)"() -> ("Value"=w510:i32)  [unwired: 2 in, 2 out]
        n552 = Subtract(x=w504, y=2) -> (x-y=w506:i32)
        n553 = Less?(x=w510, y=w506) -> (x < y?=w508:bool)
        n554 = Greater Than 0?(x=w510) -> (x > 0?=w507:bool)
        n555 = And(x=w507, y=w508) -> (x .and. y?=w509:bool)
        n556 = case shown="True" w509 {
          tunnel: w510 -> [_ w518]
          frame False {
          }
          frame True {
            n557 = Decrement(x=w518) -> (x-1=w522:i32)
            n558 = local read "Flatten Element Array"() -> (w513:string[])
            n559 = property on="Multicolumn Listbox" class="MCListbox (strict)"() -> ("ItemNames"=w529:string[][])  [unwired: 2 in, 2 out]
            n560 = Increment(x=w518) -> (x+1=w521:i32)
            n561 = Delete From Array(array=w529, index (row)=w522) -> (deleted portion=w526:string[], array with subset deleted=w528:string[][])  [unwired: 2 in]
            n562 = Delete From Array(array=w528, index (row)=w522) -> (deleted portion=w524:string[], array with subset deleted=w527:string[][])  [unwired: 2 in]
            n563 = Quotient & Remainder(x=w518, y=2) -> (floor(x/y)=w515:i32)  [unwired: 1 out]
            n564 = Insert Into Array(array=w527, index (row)=w521, new element=w526) -> (w525:string[][])  [unwired: 1 in]
            n565 = Increment(x=w521) -> (x+1=w520:i32)
            n566 = Delete From Array(array=w513, index=w515) -> (deleted portion=w517:string, array with subset deleted=w514:string[])  [unwired: 1 in]
            n567 = Increment(x=w515) -> (x+1=w516:i32)
            n568 = Insert Into Array(array=w525, index (row)=w520, new element=w524) -> (w523:string[][])  [unwired: 1 in]
            n569 = Insert Into Array(array=w514, index=w516, new element=w517) -> (w512:string[])
            n570 = property on="Multicolumn Listbox" class="MCListbox (strict)"("ItemNames"=w523) -> ()  [unwired: 2 in, 2 out]
            n571 = local write "Is Change?"(TRUE ("Is Change?")) -> ()
            n572 = property on="Flatten Element Array" class="Arr (strict)"("Val(Sgnl)"=w512) -> ()  [unwired: 2 in, 2 out]
            n573 = property on="Multicolumn Listbox" class="MCListbox (strict)"("Value"=w520) -> ()  [unwired: 2 in, 2 out]
          }
        }
      }
      frame 7 {
        n574 = flat-sequence {
          tunnel: [w535] -> w531
          tunnel: w531 -> [w538]
          frame #0 {
            n575 = property on="Multicolumn Listbox" class="MCListbox (strict)"("ItemNames"=string[][] [] ("Item Names")) -> ()  [unwired: 2 in, 2 out]
            n576 = local read "reference out"() -> (w535:refnum<vi>)
            n577 = invoke class="VI" method="Ctrl Val.Get"(reference=w535, "Control Name"="Stimulus Out") -> ("Get Control Value Variant"=w534:variant)  [unwired: 2 in, 3 out]
            n578 = invoke on="Sub Panel" class="SubPanel" method="Remove VI"() -> ()  [unwired: 3 in, 3 out]
            n579 = Variant To Data(Variant=w534) -> (data=w533:T1)  [unwired: 2 in, 1 out]
            n580 = local write "Stimulus"(w533) -> ()
          }
          frame #1 {
            n581 = call "CRYGet Boolean Reference.vi"("Label Name"="stop", "VI Refnum"=w538) -> ("Boolean Ref"=w540:refnum<vi>)  [unwired: 7 in, 2 out]
            n582 = property class="Bool"(reference=w540, "Val(Sgnl)"=TRUE ("Visible")) -> ()  [unwired: 1 in, 2 out]
          }
          frame #2 {
            n583 = local read "Flatten Element Array"() -> (w544:string[])
            n584 = control-ref of="Multicolumn Listbox"() -> (w542:refnum<vi>)
            n585 = global read "CRYStimulus Global.vi" "Flatten Element"() -> (w543:string)
            n586 = Array Size(array=w544) -> (size(s)=w546:i32)
            n587 = Equal To 0?(x=w546) -> (x = 0?=w545:bool)
            n588 = call "CRYStimulus Table Insert.vi"("Insert"=w545, "Stimulus TableRef"=w542, "Flatten Stimulus Setup String"=w543) -> ()  [unwired: 9 out]
            n589 = case shown="True" w545 {
              tunnel: w544 -> [w550 w553]
              tunnel: w543 -> [w549 w552]
              tunnel: [w547 w551] -> w541
              frame False {
                n590 = Replace Array Subset(array=w550, new element=w549, index=0) -> (w547:string[])
              }
              frame True {
                n591 = Insert Into Array(array=w553, index=0, new element=w552) -> (w551:string[])
              }
            }
            n592 = property on="Flatten Element Array" class="Arr (strict)"("Val(Sgnl)"=w541) -> ()  [unwired: 2 in, 2 out]
          }
          frame #3 {
            w556 = TRUE ("Visible")
            n593 = local write "Is Change?"(TRUE ("Is Change?")) -> ()
            n594 = property on="Table Tab" class="TabCtl (strict)"("Visible"=w556) -> ()  [unwired: 2 in, 2 out]
            n595 = property on="ViewTable" class="Bool"("Visible"=FALSE) -> ()  [unwired: 2 in, 2 out]
            n596 = property on="Is SubPan?" class="Bool (strict)"("Value"=FALSE ("Is SubPan?")) -> ()  [unwired: 2 in, 2 out]
            n597 = property on="View Edit" class="Bool"("Visible"=w556, "DisabledEnum"=T12."Enabled" ("Disabled")) -> ()  [unwired: 2 in, 2 out]
          }
        }
        n598 = property on="Remove" class="Bool"("DisabledEnum"=T12."Disabled and Grayed Out" ("Disabled")) -> ()  [unwired: 2 in, 2 out]
      }
      frame 8 {
        n599 = stacked-sequence {
          frame #0 {
            n600 = property on="Is SubPan?" class="Bool (strict)"() -> ("Value"=w560:bool)  [unwired: 2 in, 2 out]
            n601 = case shown="False" w560 {
              frame False {
                n602 = flat-sequence {
                  frame #0 {
                    w561 = FALSE ("Visible")
                    n603 = property on="Table Tab" class="TabCtl (strict)"("Visible"=w561) -> ()  [unwired: 2 in, 2 out]
                    n604 = property on="ViewTable" class="Bool"("Visible"=TRUE) -> ()  [unwired: 2 in, 2 out]
                    n605 = property on="Is SubPan?" class="Bool (strict)"("Value"=TRUE ("Is SubPan?")) -> ()  [unwired: 2 in, 2 out]
                    n606 = property on="View Edit" class="Bool"("Visible"=w561) -> ()  [unwired: 2 in, 2 out]
                  }
                  frame #1 {
                    n607 = global read "CRYRef nums global.vi" "Stimulus Sub VI ref"() -> (w564:refnum<vi>)
                    n608 = property class="VI"(reference=w564, "FP.Behavior"=T13."Default" ("Front Panel Window:Behavior")) -> (reference out=w567:refnum<vi>)  [unwired: 1 in, 1 out]
                    n609 = invoke class="VI" method="Run VI"(reference=w567, "Wait until done"=FALSE ("Wait Until Done")) -> (reference out=w568:refnum<vi>)  [unwired: 3 in, 4 out]
                    n610 = local write "reference out"(w568) -> ()
                    n611 = invoke on="Sub Panel" class="SubPanel" method="Insert VI"("VI Ref"=w568) -> ()  [unwired: 3 in, 4 out]
                  }
                }
              }
              frame True {
              }
            }
          }
          frame #1 {
            n612 = local read "reference out"() -> (w570:refnum<vi>)
            n613 = local read "Stimulus"() -> (w571:T1)
            n614 = call "CRYGet String Reference.vi"("Label Name"="Stimulus Change", "VI Refnum"=w570) -> ("String Ref Out"=w573:refnum<vi>)  [unwired: 9 out]
            n615 = call "CRYFlatten Stimulus.vi"("Stimulus"=w571) -> ("Flatten Stimulus String"=w572:string)  [unwired: 10 out]
            n616 = property class="Str"(reference=w573, "Val(Sgnl)"=w572) -> ()  [unwired: 1 in, 2 out]
          }
        }
      }
      frame 9 {
        n617 = flat-sequence {
          tunnel: [w588] -> w582
          tunnel: [w584] -> w574
          tunnel: [w594] -> w581
          tunnel: [w593] -> w580
          tunnel: w582 -> [w593]
          tunnel: w583 -> [w592]
          tunnel: w577 -> [w590]
          tunnel: [w589] -> w575
          tunnel: w574 -> [w589]
          tunnel: w581 -> [w598]
          tunnel: w580 -> [w597]
          tunnel: [w596] -> w576
          tunnel: w575 -> [w596]
          tunnel: w576 -> [w600]
          frame #0 {
            n618 = local read "Proper VI No"() -> (w584:i32)
            n619 = Build Array(w584) -> (w587:i32[])
            n620 = call "CRYGet Curve Library Data Name.vi"("nData"=w587, "sAction"="GetNamebyStep" ("sOption"), "Type"=enum16{"Curves", "Values", "Results", "WFM"}."WFM") -> ("sNames"=w588:string[])  [unwired: 5 in, 3 out]
          }
          frame #1 {
            n621 = call "CRYFlatten Stimulus.vi"("Stimulus"=w592) -> ("Flatten Stimulus String"=w591:string)  [unwired: 10 in]
            n622 = call "CRYReplace Stimulus Curve Name.vi"("Setup in"=w590, "Step Setup In"=w591, "Type In"="AddStep" ("Type")) -> ("Inserted Names Out"=w594:string[])  [unwired: 8 in]
          }
          frame #2 {
            n623 = call "CRYReplace Curve Name of Steps.vi"("Step Category"="Stimulus", "New Name"=w598, "Old Name"=w597) -> ()  [unwired: 8 in, 1 out]
          }
          frame #3 {
            n624 = global read "CRYStepSetup Global.vi" "Load from AddStep"() -> (w601:bool)
            n625 = local write "Add Lib"(FALSE ("Add Lib")) -> ()
            n626 = case shown="True" w601 {
              tunnel: w600 -> [_ w604]
              frame False {
              }
              frame True {
                n627 = global write "CRYStepSetup Global.vi" "Load from AddStep"(FALSE ("Load from AddStep")) -> ()
                n628 = call "CRYStepData Manipulate.vi"("sAction"="Backup", "StepNo."=w604) -> ()  [unwired: 10 in]
              }
            }
          }
        }
        n629 = local read "Stimulus"() -> (w583:T1)
        n630 = call "CRYGet Current TS Steps.vi"() -> ("SelectStepNumber in Tree"=w579:i32, "Steps"=w578:T11[])  [unwired: 1 in, 9 out]
        n631 = Index Array(array=w578, index=w579) -> (element=w577:T11)
      }
      frame 10 {
        n632 = flat-sequence {
          frame #0 {
            n633 = global read "CRYMainGlobal.vi" "Access Level"() -> (w606:enum16{"Engineer", "Technician", "Operator"})
            n634 = case shown="\"Technician\", Default" w606 {
              frame "Engineer" {
                n635 = flat-sequence {
                  tunnel: [w610] -> w609
                  tunnel: [w623] -> w608
                  tunnel: [w627] -> w607
                  tunnel: w609 -> [w625]
                  tunnel: w608 -> [w652]
                  tunnel: w607 -> [w656]
                  frame #0 {
                    n636 = local read "Flatten Element Array"() -> (w613:string[])
                    n637 = global read "CRYStimulus Global.vi" "Flatten Element"() -> (w614:string)
                    n638 = Array Size(array=w613) -> (size(s)=w611:i32)
                    n639 = Equal To 0?(x=w611) -> (x = 0?=w612:bool)
                    n640 = case shown="False" w612 {
                      tunnel: w613 -> [w618 w621]
                      tunnel: w614 -> [w617 w620]
                      tunnel: [w615 w619] -> w610
                      frame False {
                        n641 = Replace Array Subset(array=w618, new element=w617, index=0) -> (w615:string[])
                      }
                      frame True {
                        n642 = Insert Into Array(array=w621, index=0, new element=w620) -> (w619:string[])
                      }
                    }
                  }
                  frame #1 {
                    n643 = property on="Is First" class="Bool (strict)"() -> ("Value"=w632:bool)  [unwired: 2 in, 2 out]
                    n644 = property on="Is SubPan?" class="Bool (strict)"() -> ("Value"=w631:bool)  [unwired: 2 in, 2 out]
                    n645 = local read "Stimulus"() -> (w635:T1)
                    n646 = local read "Signal Type Name"() -> (w640:string)
                    n647 = Not(x=w632) -> (.not. x?=w633:bool)
                    n648 = local read "Channel Out"() -> (w639:u32)
                    n649 = And(x=w631, y=w633) -> (x .and. y?=w634:bool)
                    n650 = case shown="False" w634 {
                      tunnel: w635 -> [w645 w647]
                      tunnel: [w645 w646] -> w641
                      frame False {
                      }
                      frame True {
                        n651 = local read "reference out"() -> (w649:refnum<vi>)
                        n652 = invoke class="VI" method="Ctrl Val.Get"(reference=w649, "Control Name"="Stimulus Out") -> ("Get Control Value Variant"=w648:variant)  [unwired: 2 in, 3 out]
                        n653 = Variant To Data(type=w647, Variant=w648) -> (data=w646:T1)  [unwired: 1 in, 1 out]
                      }
                    }
                    n654 = property on="Duration(s)" class="DigNum (strict)"() -> ("Value"=w637:dbl)  [unwired: 2 in, 2 out]
                    n655 = property on="Custom Stimulus Name" class="Str"() -> ("Value"=w638:string)  [unwired: 2 in, 2 out]
                    n656 = property on="Apply EQ" class="Bool (strict)"() -> ("Value"=w636:bool)  [unwired: 2 in, 2 out]
                    n657 = Bundle By Name(cluster=w641, "Flatten Element Array"=w625, "Duration(s)"=w637, "CustomStimulusName"=w638, "ApplyEQ"=w636, "Channel Out"=w639, "Signal Type Name"=w640) -> (w624:T1)
                    n658 = local read "Proper VI No"() -> (w626:i32)
                    n659 = call "CRYFlatten Stimulus.vi"("Stimulus"=w624) -> ("Flatten Stimulus String"=w623:string)  [unwired: 10 out]
                    n660 = Build Array(w626) -> (w628:i32[])
                    n661 = call "CRYGet Curve Library Data Name.vi"("nData"=w628, "sAction"="GetNamebyStep" ("sOption"), "Type"=enum16{"Curves", "Values", "Results", "WFM"}."WFM") -> ("sNames"=w627:string[])  [unwired: 5 in, 3 out]
                    n662 = call "CRYPreUpdate Sequence.vi"("EventName"="SequenceUpdate", "Proper VI No"=w626, "Project View Step Name Identifier Arg1"="", "Step flattened Arg2"=w623, "AllChangeFlg"=TRUE ("Name/Identifier")) -> ()  [unwired: 11 in]
                  }
                  frame #2 {
                    n663 = local read "Calibration setup In"() -> (w655:string)
                    n664 = local read "Hardware setup In"() -> (w654:string)
                    n665 = call "CRYGet Current TS Steps.vi"() -> ("SelectStepNumber in Tree"=w657:i32, "Steps"=w658:T11[])  [unwired: 1 in, 9 out]
                    n666 = Index Array(array=w658, index=w657) -> (element=w653:T11)
                    n667 = Bundle By Name(cluster=w653, "Seq setup flattened"=w652) -> (w651:T11)
                    n668 = call "CRYReplace Stimulus Curve Name.vi"("Setup in"=w653, "Step Setup In"=w652, "Type In"="StepOK" ("Type")) -> ("Inserted Names Out"=w660:string[])  [unwired: 8 in]
                    n669 = call "CRYStimulus.vi"("Setup in"=w651, "Hardware in"=w654, "Calibration in"=w655) -> ()  [unwired: 8 in, 5 out]
                    n670 = call "CRYReplace Curve Name of Steps.vi"("Step Category"="Stimulus", "New Name"=w660, "Old Name"=w656) -> ()  [unwired: 8 in, 1 out]
                  }
                }
              }
              frame "Technician", Default {
                n671 = call "CRYGet Error Message.vi"("Kind"="Step Setup") -> ("Window Title"=w664:string)  [unwired: 5 in, 5 out]
                n672 = call "CRYGet Access Level Message.vi"("sAction"="OK") -> ("Multibyte string"=w666:string)  [unwired: 10 in]
                n673 = call "CRYMessage Dialog.vi"("Window Title"=w664, "YesNoCancel"=T14."OK", "Message Content"=w666) -> ()  [unwired: 7 in, 2 out]
              }
            }
          }
          frame #1 {
            n674 = local write "stop"(TRUE ("stop")) -> ()
            n675 = local write "OK"(FALSE ("OK")) -> ()
          }
        }
      }
      frame 11 {
        n676 = flat-sequence {
          frame #0 {
            n677 = local read "Proper VI No"() -> (w670:i32)
            n678 = call "CRYStepData Manipulate.vi"("sAction"="Restore", "StepNo."=w670) -> ()  [unwired: 10 in]
          }
          frame #1 {
            n679 = local write "Cancel"(FALSE ("Cancel")) -> ()
          }
        }
        n680 = local write "stop"(TRUE ("stop")) -> ()
      }
    }
    n681 = global read "CRYMain Sub Window Global.vi" "gStop"() -> (w54:bool)
    n682 = global read "CRYMainGlobal.vi" "STOP"() -> (w66:bool)
    n683 = local read "Is SubPan?"() -> (w61:bool)
    n684 = Unbundle By Name(w45) -> ("start"=w65:bool)
    n685 = Compound Arithmetic op=OR(w54, "stop", w66) -> (w63:bool)
    n686 = Not(x=w65) -> (.not. x?=w64:bool)
    n687 = And(x=w63, y=w64) -> (x .and. y?=w48:bool)
    n688 = And(x=w48, y=w61) -> (x .and. y?=w60:bool)
    n689 = case shown="True" w60 {
      frame False {
      }
      frame True {
        n690 = flat-sequence {
          frame #0 {
            n691 = invoke on="Sub Panel" class="SubPnl" method="Remove VI"() -> ()  [unwired: 3 in, 3 out]
          }
          frame #1 {
            n692 = local read "reference out"() -> (w88:refnum<vi>)
            n693 = property class="VI"(reference=w88, "Front Panel Window:Open"=FALSE ("Front Panel.Open")) -> (reference out=w85:refnum<vi>)  [unwired: 1 in, 1 out]
            n694 = call "CRYGet Boolean Reference.vi"("Label Name"="stop", "VI Refnum"=w85) -> ("Boolean Ref"=w84:refnum<vi>)  [unwired: 7 in, 2 out]
            n695 = property class="Bool"(reference=w84, "Val(Sgnl)"=TRUE ("Front Panel.Open")) -> ()  [unwired: 1 in, 2 out]
          }
        }
      }
    }
    n696 = case shown="True" w63 {
      frame False {
      }
      frame True {
        n697 = local write "Play"(FALSE ("Play")) -> ()
      }
    }
  }
  n698 = flat-sequence {
    tunnel: w1 -> [_]
    frame #0 {
      n699 = control-ref of="This VI"() -> (w894:refnum<vi>)
      n700 = call "CRYWork Before Step Close.vi"("StepVI Ref"=w894) -> ()  [unwired: 11 in]
    }
    frame #1 {
      n701 = local write "EndFlag"(TRUE ("EndFlag")) -> ()
    }
  }
